vi "GDSIconEditor_GlyphEditorDialog.vi"(8 "error in (no error)":errorcluster, 11 "IconInfo":T3={"HeaderIcon"=[], "RowStart(0)"=0, "ImageRows(32)"=32, "FrameThickness(1)"=1, "FrameColor"=0, "IconTextDataType"={"Text"="", "Allow Only Capital Chars"=FALSE, "Compression"=enum."Auto", "Alignment"=enum."Center"}, "BodyTextColor"=0, "BodyBackgroundColor"=0, "BodyIconHeight"=0, "BodyIconWidth"=0, "HeaderBackgroundColor"=0, "BodyIcon"=[[0, 0, 0, 0, 0, 0, 0, 0, 0, 0, 255, 255, 0, 0, 255, 0, 0, 0, 255, 0, 0, 0, 0, 0, 0, 0, 0, 0, 0, 0], [0, 0, 0, 0, 0, 0, 0, 0, 0, 255, 0, 0, 255, 0, 255, 0, 0, 0, 255, 0, 0, 0, 0, 0, 0, 0, 0, 0, 0, 0], [0, 0, 0, 0, 0, 0, 0, 0, 0, 255, 255, 255, 255, 0, 255, 0, 0, 0, 255, 0, 0, 0, 0, 0, 0, 0, 0, 0, 0, 0], [0, 0, 0, 0, 0, 0, 0, 0, 0, 255, 0, 0, 255, 0, 255, 0, 0, 0, 255, 0, 0, 0, 0, 0, 0, 0, 0, 0, 0, 0], [0, 0, 0, 0, 0, 0, 0, 0, 0, 255, 0, 0, 255, 0, 255, 255, 255, 0, 255, 255, 255, 0, 0, 0, 0, 0, 0, 0, 0, 0], [0, 0, 255, 0, 0, 0, 255, 0, 0, 255, 255, 0, 0, 255, 0, 0, 255, 0, 255, 255, 0, 255, 255, 0, 0, 0, 255, 255, 0, 0], [0, 255, 0, 255, 0, 255, 0, 255, 0, 255, 0, 255, 0, 255, 255, 0, 255, 0, 255, 0, 0, 255, 0, 255, 0, 255, 0, 0, 0, 0], [0, 255, 0, 0, 0, 255, 0, 255, 0, 255, 255, 0, 0, 255, 0, 255, 255, 0, 255, 255, 0, 255, 255, 0, 0, 0, 255, 0, 0, 0], [0, 255, 0, 255, 0, 255, 0, 255, 0, 255, 0, 255, 0, 255, 0, 0, 255, 0, 255, 0, 0, 255, 0, 255, 0, 0, 0, 255, 0, 0], [0, 0, 255, 0, 0, 0, 255, 0, 0, 255, 0, 255, 0, 255, 0, 0, 255, 0, 255, 255, 0, 255, 0, 255, 0, 255, 255, 0, 0, 0], [0, 255, 0, 0, 0, 255, 0, 0, 255, 0, 0, 255, 0, 255, 0, 0, 255, 0, 255, 255, 0, 0, 255, 0, 0, 255, 255, 255, 0, 255], [255, 0, 255, 0, 255, 0, 255, 0, 255, 255, 0, 255, 0, 255, 255, 0, 255, 0, 255, 0, 0, 255, 0, 255, 0, 0, 255, 0, 0, 255], [255, 0, 0, 0, 255, 0, 255, 0, 255, 0, 255, 255, 0, 255, 0, 255, 255, 0, 255, 255, 0, 255, 0, 0, 0, 0, 255, 0, 0, 255], [255, 0, 255, 0, 255, 0, 255, 0, 255, 0, 0, 255, 0, 255, 0, 0, 255, 0, 255, 0, 0, 255, 0, 255, 0, 0, 255, 0, 0, 255], [0, 255, 0, 0, 0, 255, 0, 0, 255, 0, 0, 255, 0, 255, 0, 0, 255, 0, 255, 255, 0, 0, 255, 0, 0, 0, 255, 0, 0, 255], [0, 0, 0, 0, 0, 0, 0, 0, 0, 0, 0, 0, 0, 0, 255, 0, 0, 0, 0, 0, 0, 0, 0, 0, 0, 0, 0, 0, 0, 0], [0, 0, 0, 0, 0, 0, 0, 0, 0, 0, 0, 0, 0, 255, 0, 0, 0, 0, 0, 0, 0, 0, 0, 0, 0, 0, 0, 0, 0, 0], [0, 0, 0, 0, 0, 0, 0, 0, 0, 0, 0, 0, 0, 255, 255, 0, 0, 0, 0, 0, 0, 0, 0, 0, 0, 0, 0, 0, 0, 0], [0, 0, 0, 0, 0, 0, 0, 0, 0, 0, 0, 0, 0, 255, 0, 255, 0, 0, 0, 0, 0, 0, 0, 0, 0, 0, 0, 0, 0, 0], [0, 0, 0, 0, 0, 0, 0, 0, 0, 0, 0, 0, 0, 0, 255, 0, 0, 0, 0, 0, 0, 0, 0, 0, 0, 0, 0, 0, 0, 0], [0, 0, 0, 0, 0, 0, 0, 0, 0, 0, 0, 0, 0, 0, 0, 0, 0, 0, 0, 0, 0, 0, 0, 0, 0, 0, 0, 0, 0, 0], [0, 0, 0, 0, 0, 0, 0, 0, 0, 0, 0, 0, 0, 0, 0, 0, 0, 0, 0, 0, 0, 0, 0, 0, 0, 0, 0, 0, 0, 0]], "Offset"={"X"=0, "Y"=0}, "CurrentIcon"={"BgIcon"=[], "BgIconOffset"={"X"=0, "Y"=0}, "BgIconMask"=[], "ColorsOkayforiconToBeOnTopOf"=[]}} {"HeaderIcon" format="%x"}) -> (0 "error out":errorcluster, 1 "Icon exist":bool, 2 "CurrentIcon":T2, 3 "Cancelled":bool, 5 "Offset":cluster{"X":i32, "Y":i32}, 7 "BodyIcon":u8[][](array[numeric]))   [LabVIEW 2020]
uses:
  <resource>/Framework/Providers/Open_GDS/ClassProviders/Common/IconEditor/private/GDSIconEditor_IconDialog_Input.vi
  <resource>/Framework/Providers/Open_GDS/ClassProviders/Common/LvIcon_class/subvis/GDSLvIcon_TextDataType.ctl
  <resource>/Framework/Providers/Open_GDS/ClassProviders/Common/LvIcon_class/GDSLvIcon_WordCompressionType.ctl
  <resource>/Framework/Providers/Open_GDS/ClassProviders/Common/LvIcon_class/GDSLvIcon_TextAlignment.ctl
  <vilib>/picture/picture.llb/imagedata.ctl
  <vilib>/Utility/miscctls.llb/LVPoint32TypeDef.ctl
  <vilib>/Utility/miscctls.llb/LVPointTypeDef.ctl
  <vilib>/Utility/miscctls.llb/LVPositionTypeDef.ctl
panel:
  in  "Positon":T1(ring)
  in  "Relative to Error terminals":bool
  out "_IconPreview 2":picture caption="Icon Preview"
  out "_After 2":picture caption="New"
  in  "Remove Configuration":bool
  in  "Add Configuration":bool
  in  "Quick selection icons":i32(listbox)
  out "_IconPreview":picture caption="Icon Preview"
  in  "FloodFillMask":bool
  out "_After":picture caption="New"
  out "_IconName":string
  out "DragIcon":picture
  out "ProductPicture":picture
  in  "_IconSearchText":string caption="Icon search text"
  in  "_Manage":bool
  in  "_Folders":u16(ring) caption="Folders" items=["<All icons>", "C:\\Program Files (x86)\\National Instruments\\LabVIEW 2020\\resource\\Framework\\Providers\\Icons", "C:\\Program Files (x86)\\National Instruments\\LabVIEW 2020\\resource\\Framework\\Providers\\Open_GDS\\Glyphs", "C:\\Program Files (x86)\\National Instruments\\LabVIEW 2020\\resource\\Framework\\Providers\\Open_GDS\\Icons", "C:\\Users\\mikael.holmstrom\\Documents\\LabVIEW Data\\Glyphs"]
  out "Icons":picture
  in  "_HelpCreateClass":bool
  in  "_Cancel":bool
  in  "Accept":bool
  # "Drag icon into preview wndow"
  # "User arrow keys to move text,\nor drar the text to move it."
  # "User arrow keys to move text,\nor drar the text to move it."
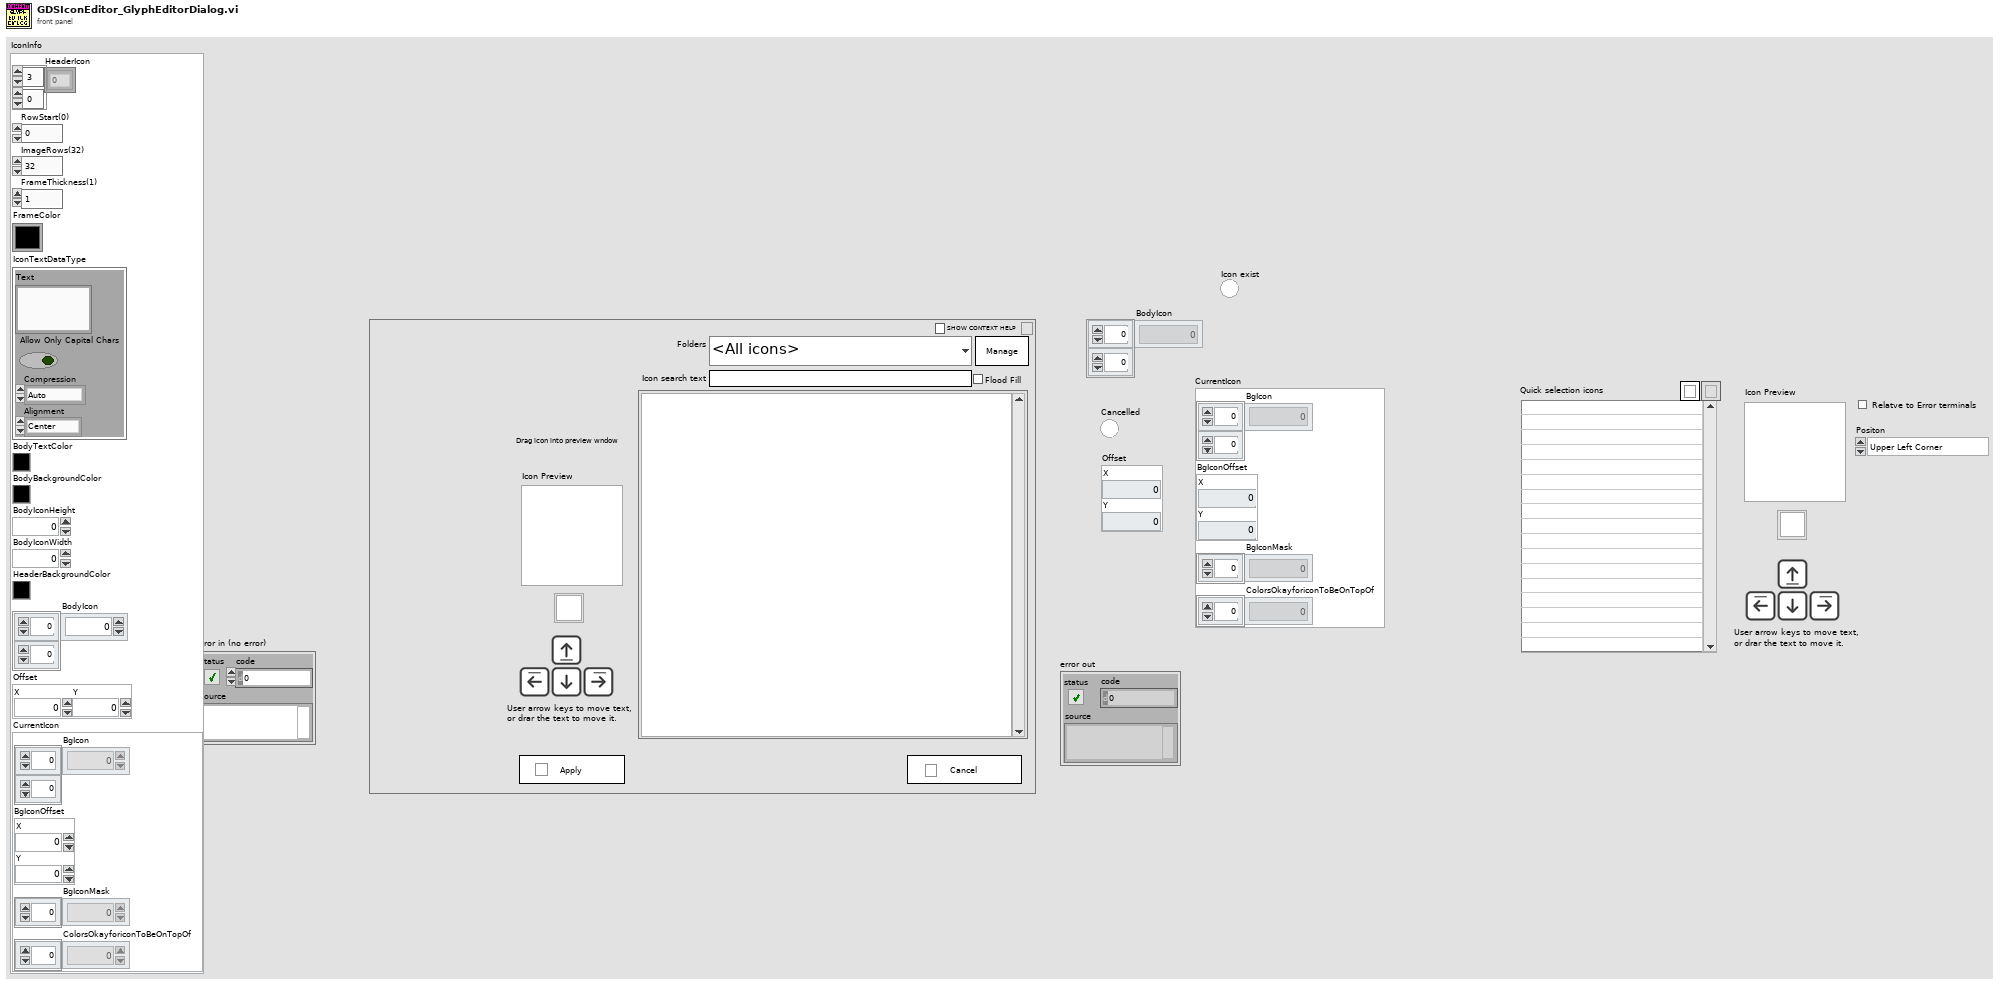
[diagram p1: front panel]
types:
  T1 = enum16{"Upper Left Corner", "Error In Terminal (Center)"}
  T2 = cluster{"BgIcon":u8[][], "BgIconOffset":cluster{"X":i32, "Y":i32}, "BgIconMask":u8[], "ColorsOkayforiconToBeOnTopOf":u8[]}
  T3 = typedef "GDSIconEditor_IconDialog_Input.vi" = cluster{"HeaderIcon":u8[][], "RowStart(0)":i32, "ImageRows(32)":i32, "FrameThickness(1)":u32, "FrameColor":u32, "IconTextDataType":T4, "BodyTextColor":u32, "BodyBackgroundColor":u32, "BodyIconHeight":i32, "BodyIconWidth":i32, "HeaderBackgroundColor":u32, "BodyIcon":u8[][], "Offset":cluster{"X":i32, "Y":i32}, "CurrentIcon":cluster{"BgIcon":u8[][], "BgIconOffset":cluster{"X":i32, "Y":i32}, "BgIconMask":u8[], "ColorsOkayforiconToBeOnTopOf":u8[]}}
  T4 = typedef "GDSLvIcon_TextDataType.ctl" = cluster{"Text":string, "Allow Only Capital Chars":bool, "Compression":T5, "Alignment":T6}
  T5 = typedef "GDSLvIcon_WordCompressionType.ctl" = enum16{"Auto", "On", "Off"}
  T6 = typedef "GDSLvIcon_TextAlignment.ctl" = enum16{"Center", "Left", "Right"}
  T7 = typedef "imagedata.ctl" = cluster{"image type":i32, "image depth":i32, "image":u8[], "mask":u8[], "colors":u32[], "Rectangle":cluster{"left":i16, "top":i16, "right":i16, "bottom":i16}}
  T8 = typedef "LVPoint32TypeDef.ctl" = cluster{"Horizontal":i32, "Vertical":i32}
  T9 = cluster{"Icons":T7[], "Folders":path[], "IconPaths":cluster{i32, "path out":path}[], "IconPos":cluster{"left":i16, "top":i16, "right":i16, "bottom":i16}[], "IconNames":string[], "DraggingIcon":bool, "DraggingText":bool, "IconSelected":i32, "IconDropped":i32, "BgIcon":u8[][], "BgIconOffset":cluster{"X":i32, "Y":i32}, "BgIconMask":u8[], "IconOut":u8[][], "ConnectorPaneHeight":i32[], "BodyIcon":u8[][], "Cancelled":bool, "StartTextDraggingPos":T8, "OldOffset":cluster{"X":i32, "Y":i32}, "TextBounds":cluster{"FirstRow":i32, "FirstColumn":i32, "LastRow":i32, "LastColumn":i32}, "Moving":bool, "Icon exist":bool, "IconInfo":T3}
  T10 = typedef "LVPointTypeDef.ctl" = cluster{"Horizontal":i16, "Vertical":i16}
  T11 = typedef "LVPositionTypeDef.ctl" = cluster{"Left":i32, "Top":i32}
  T12 = typedef "LVBoundsTypeDef.ctl" = cluster{"Width":u32, "Height":u32}
  T13 = cluster{"left":i16, "top":i16, "right":i16, "bottom":i16}
  T14 = cluster{"left":i16, "top":i16, "right":i16, "bottom":i16}[]
  T15 = typedef "LVMouseTypeDef.ctl" = cluster{"Mouse Position":cluster{"X":i32, "Y":i32}, "Mouse Modifiers":cluster{"Button Down":bool, "Shift Mod":bool, "Menu Mod":bool, "Option Mod":bool}}
  T16 = cluster{"FirstRow":i32, "FirstColumn":i32, "LastRow":i32, "LastColumn":i32}
  T17 = typedef "eventvkey.ctl" = enum16{"ASCII", "Enter", "Return", "Shift", "Ctrl", "Alt", "Cmd", "Opt", "Caps", "NumLock", "Clear", "Break", "Up", "Down", "Left", "Right", "Insert", "Delete", "Home", "End", "PageUp", "PageDown", "Escape", "Help", "Pause", "ScrollLock", "F1", "F2", "F3", "F4", "F5", "F6", "F7", "F8", "F9", "F10", "F11", "F12", "F13", "F14", "F15", "F16", "F17", "F18", "F19", "F20", "F21", "F22", "F23", "F24", "Play", "VolumeUp", "VolumeDown", "Mute", "Two Byte Char"}
  T18 = cluster{"Shift":bool, "Ctrl":bool, "Alt":bool, "Cmd":bool, "Opt":bool}
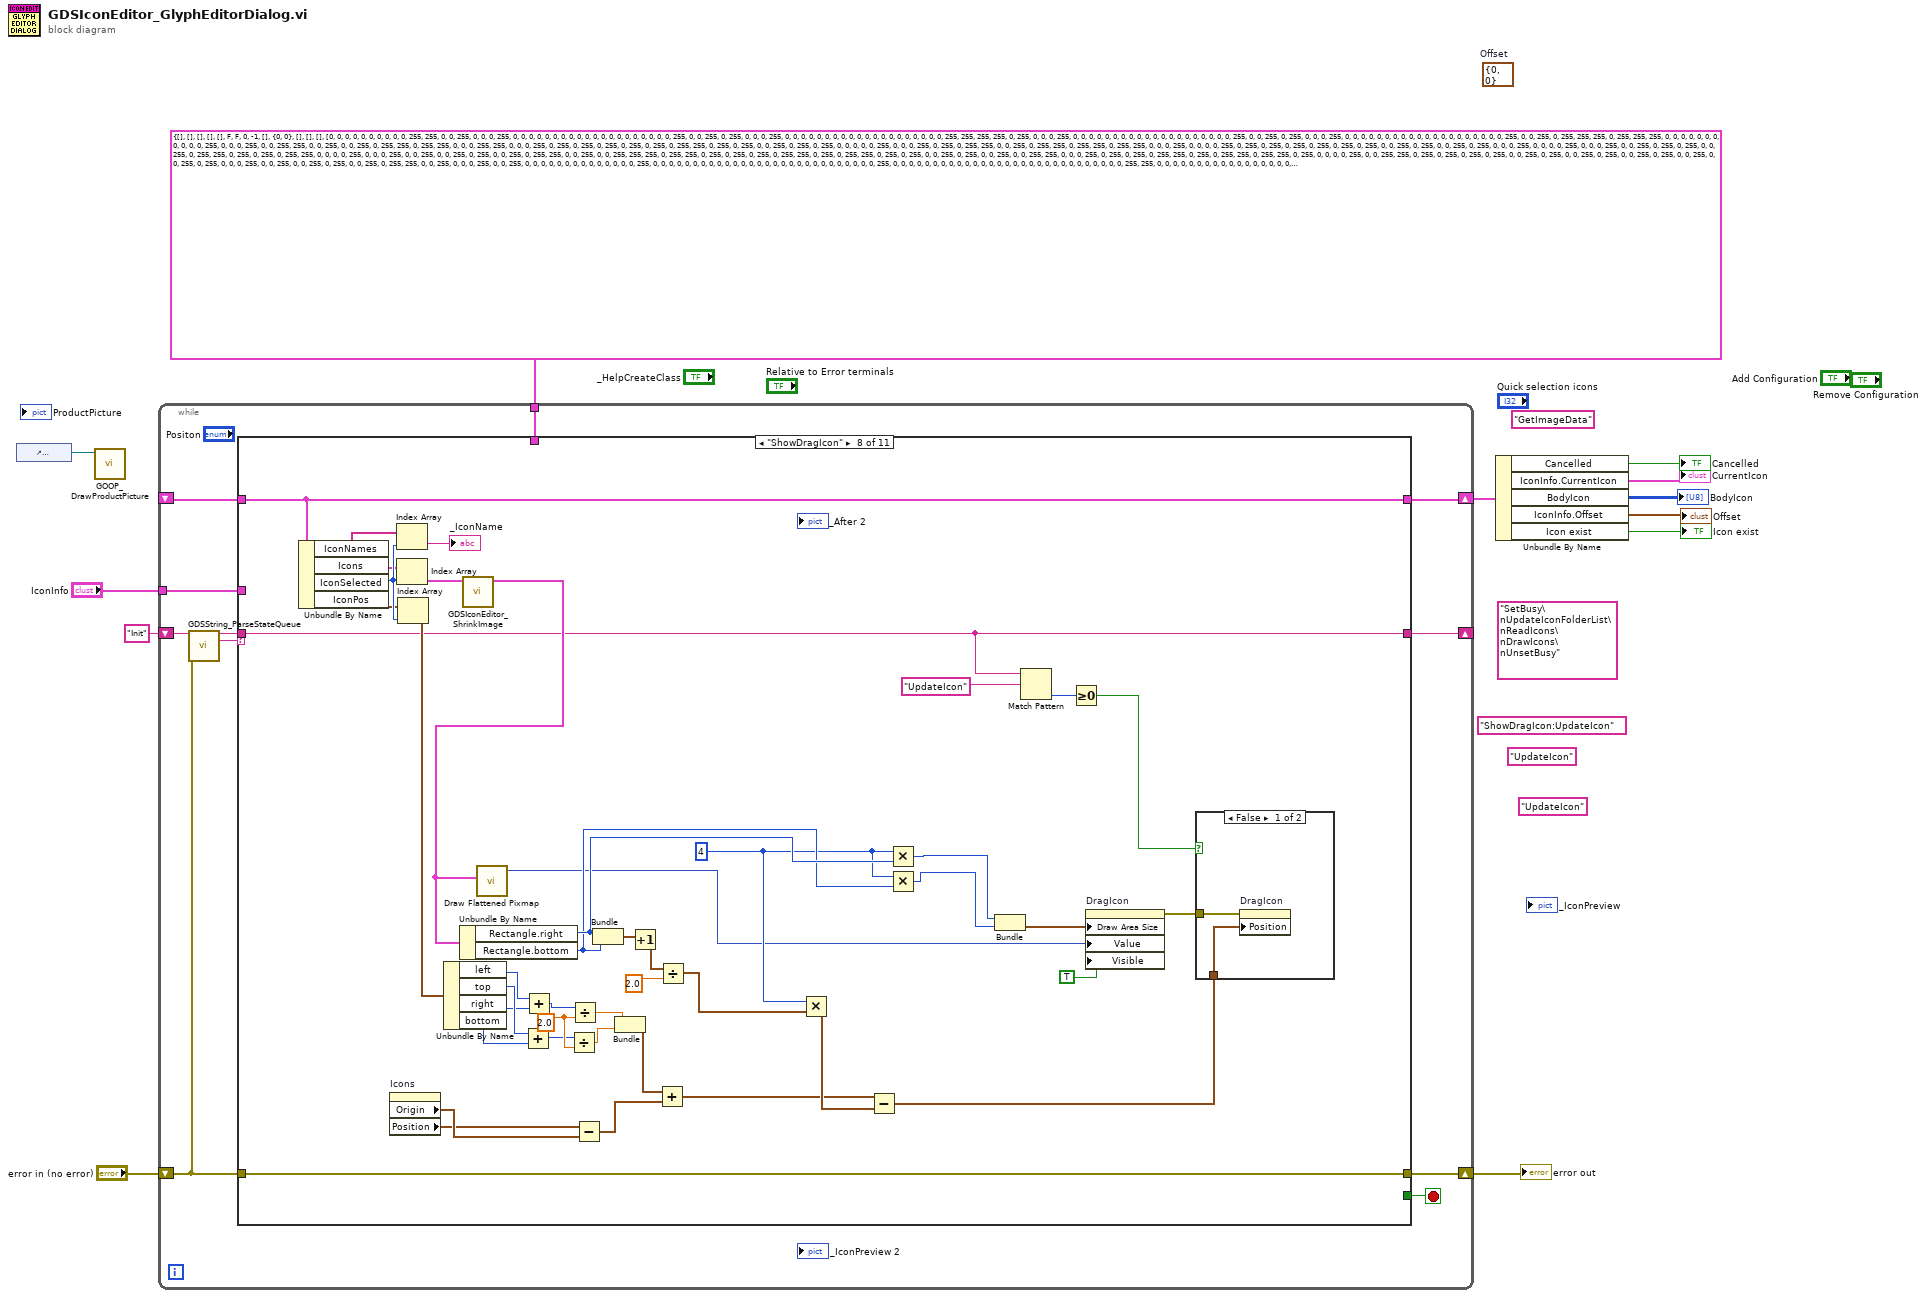
[diagram p0: block diagram]
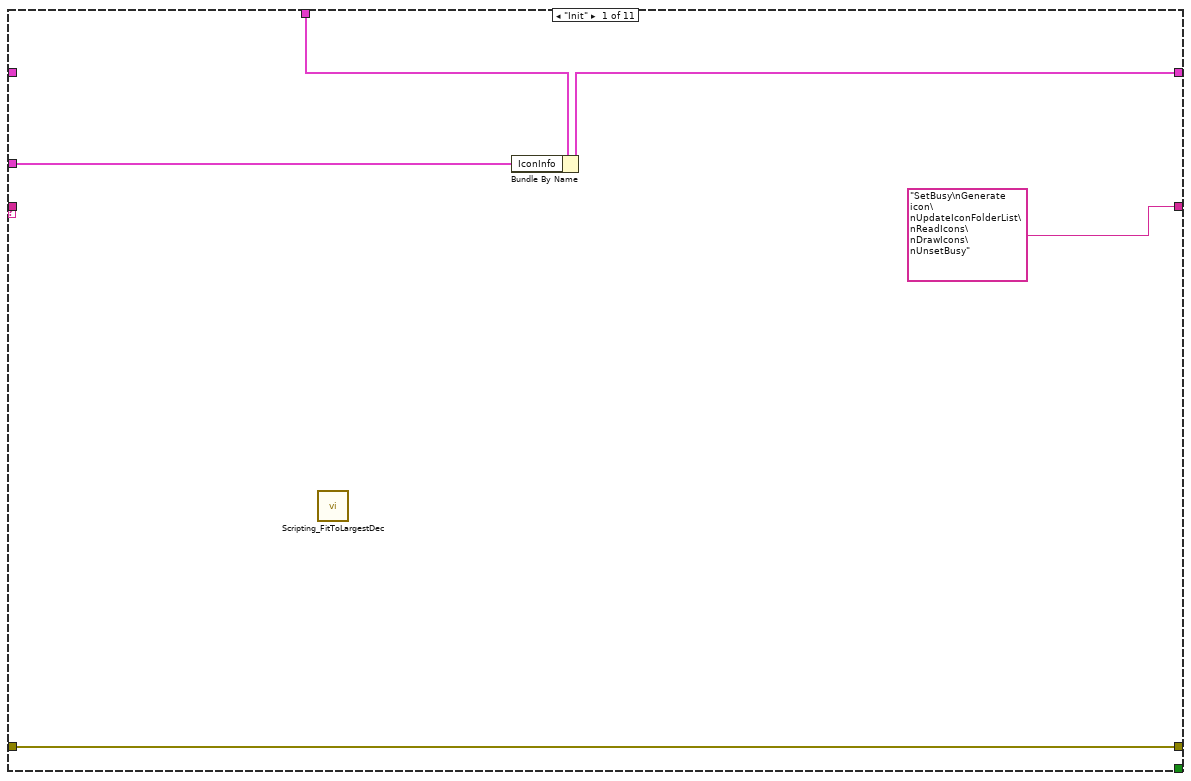
[diagram p2: hidden frame]
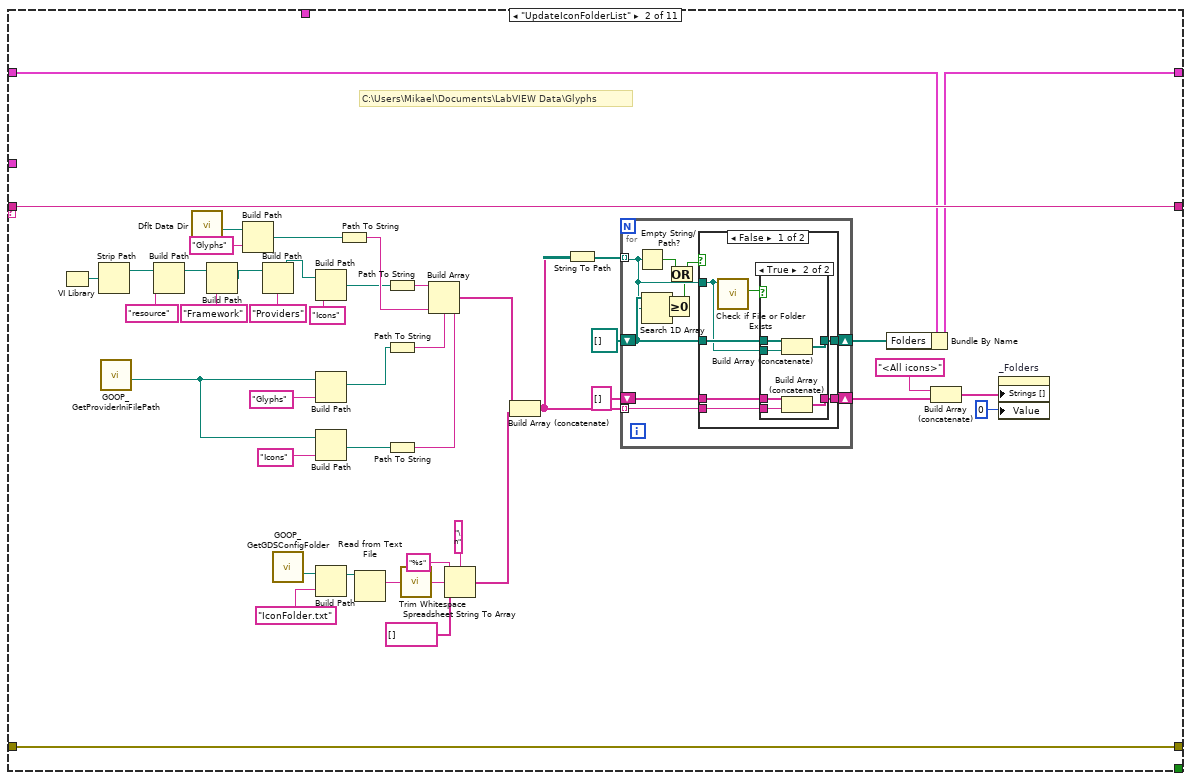
[diagram p3: hidden frame]
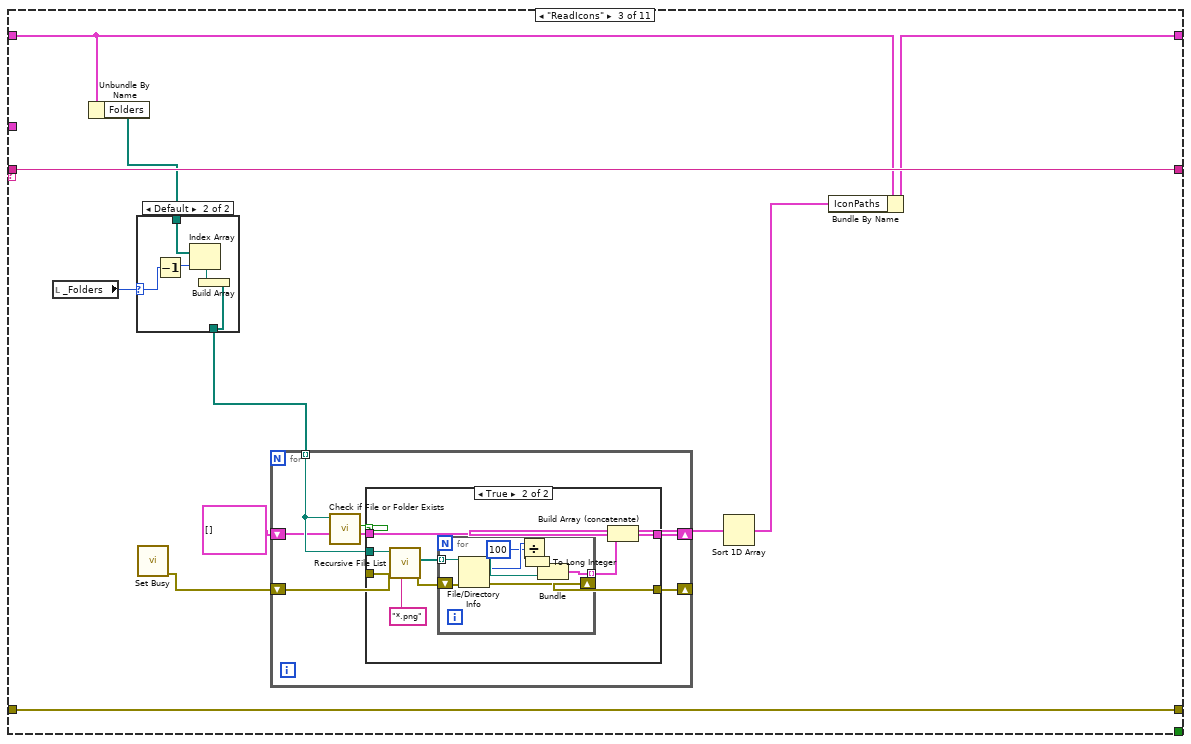
[diagram p6: hidden frame]
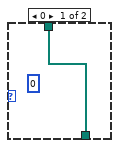
[diagram p7: hidden frame]
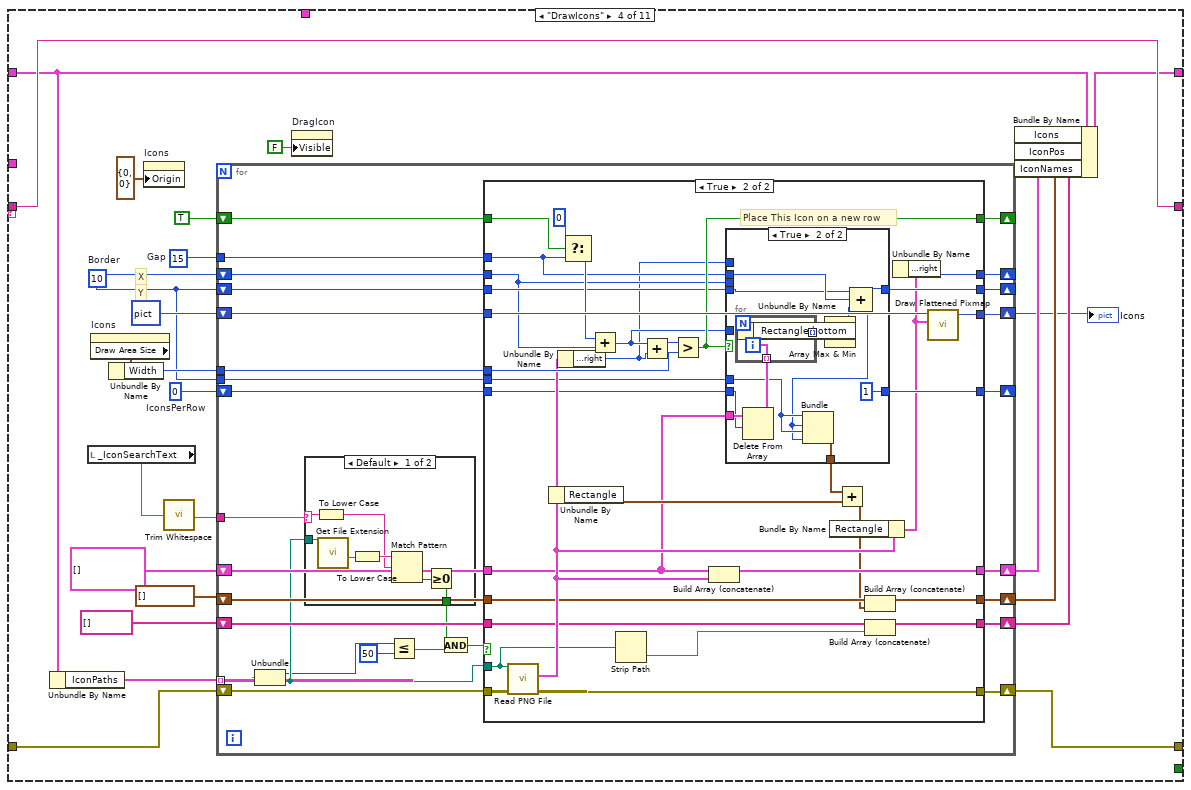
[diagram p9: hidden frame]
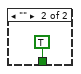
[diagram p10: hidden frame]
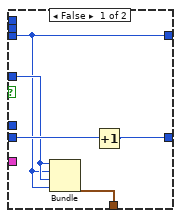
[diagram p12: hidden frame]
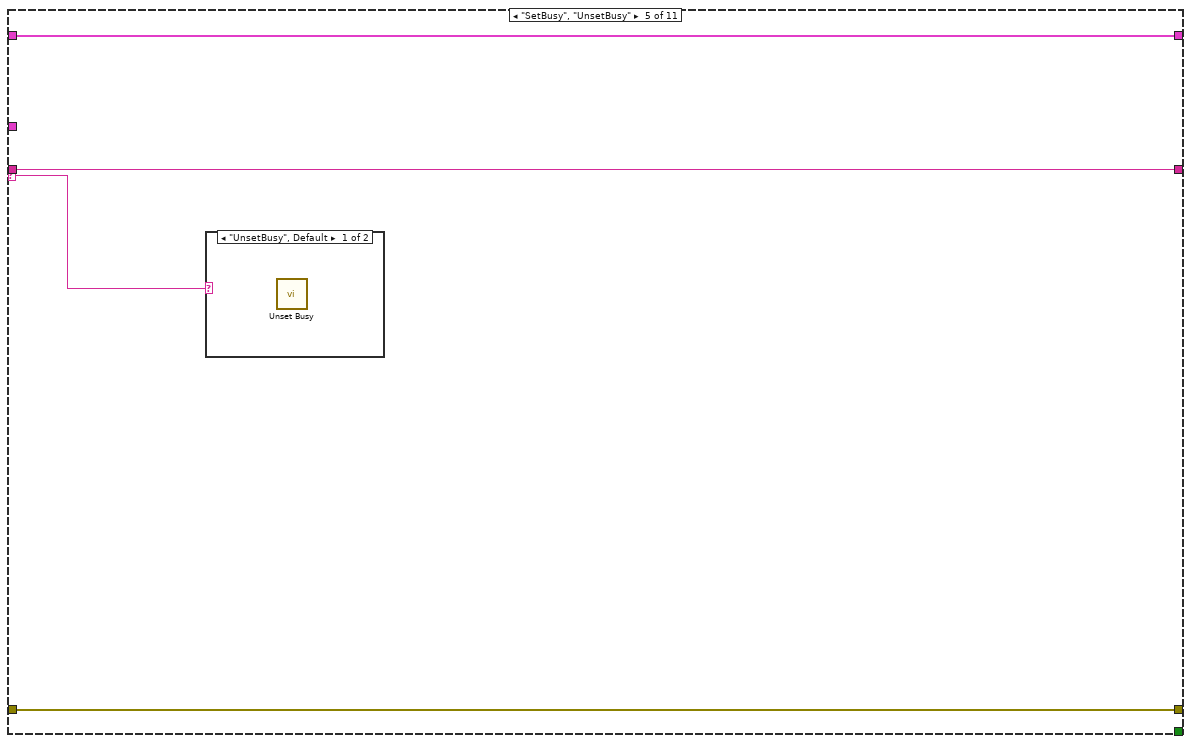
[diagram p13: hidden frame]
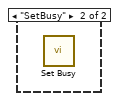
[diagram p14: hidden frame]
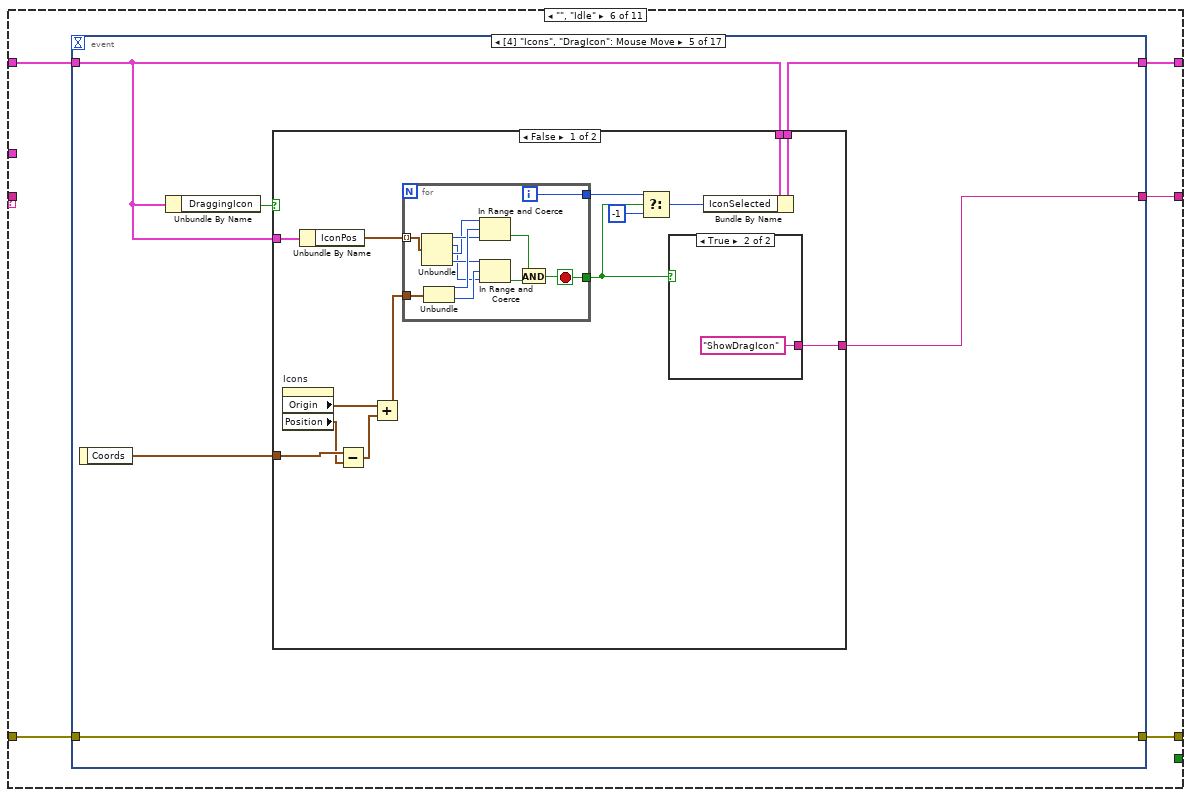
[diagram p15: hidden frame]
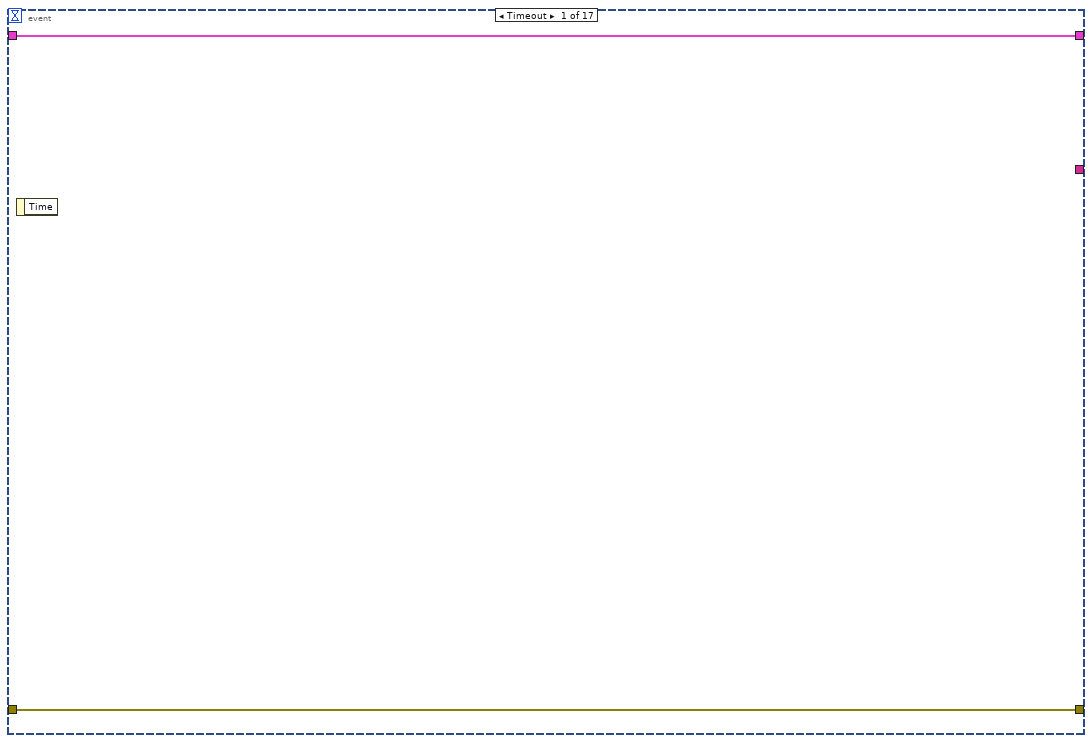
[diagram p16: hidden frame]
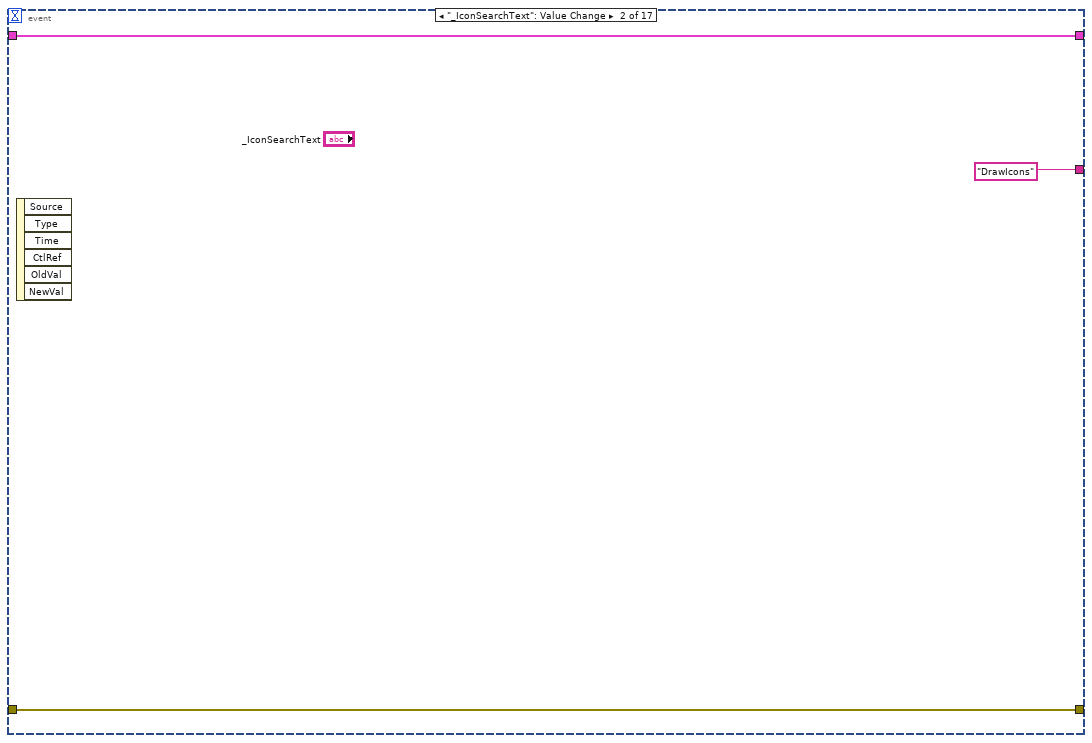
[diagram p17: hidden frame]
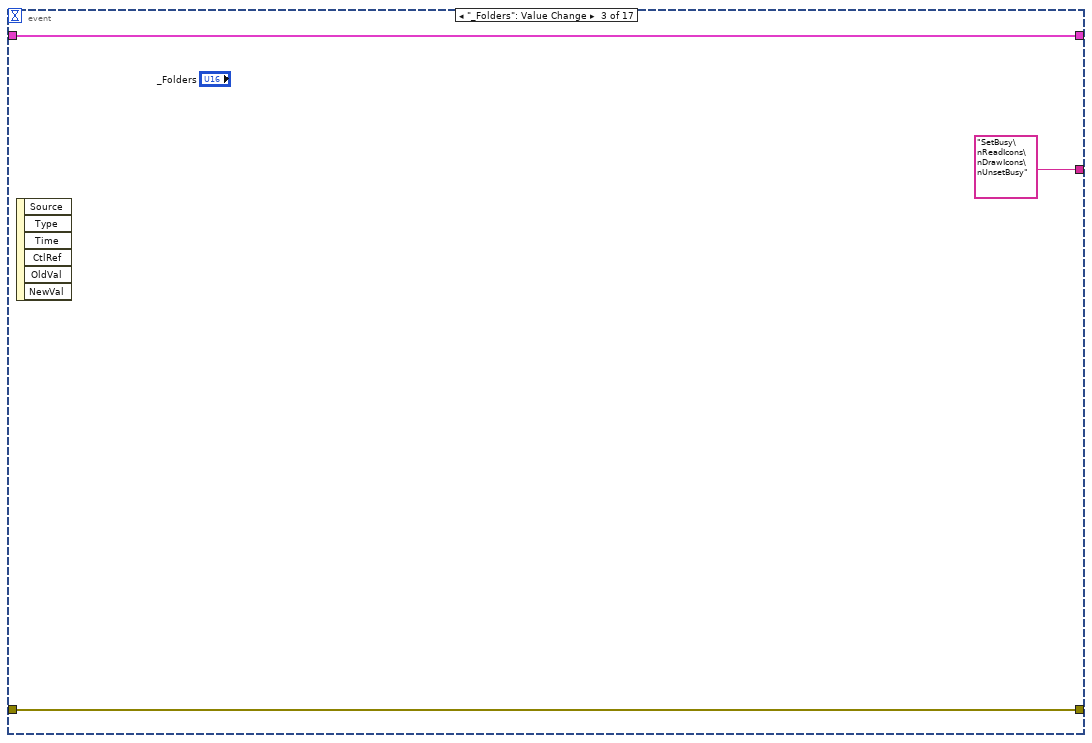
[diagram p18: hidden frame]
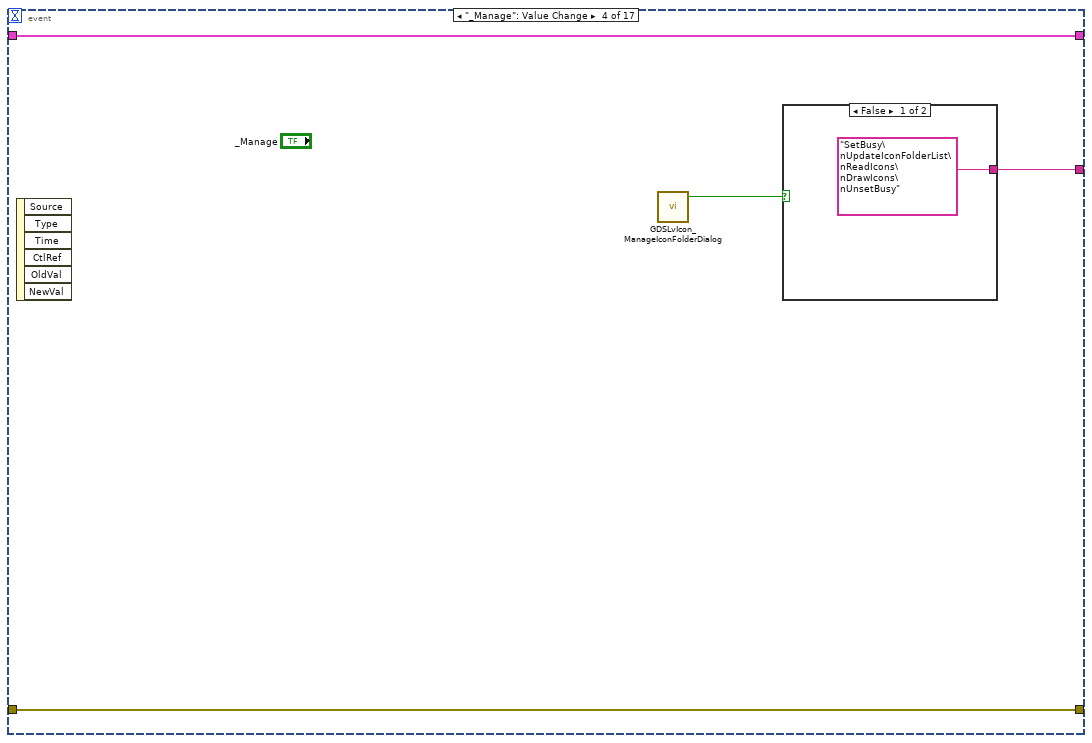
[diagram p19: hidden frame]
diagram:
  (unwired) cluster{"X":i32, "Y":i32} {"X"=0, "Y"=0}  # Offset
  (unwired) "UpdateIcon" ("y")
  (unwired) "GetImageData" ("y")
  (unwired) "ShowDragIcon:UpdateIcon" ("y")
  (unwired) "UpdateIcon" ("t")
  (unwired) "SetBusy\nUpdateIconFolderList\nReadIcons\nDrawIcons\nUnsetBusy"
  n1 = control-ref of="ProductPicture"() -> (w1:refnum<vi>)
  n2 = call <resource>:"GOOP_DrawProductPicture.vi"("ProductPictureControl"=w1) -> ()  [unwired: 10 in, 1 out]
  n3 = while {
    shift-right: [w22] -> w8
    shift-left: _ -> [w17]
    tunnel: T9 {"Icons"=[], "Folders"=[], "IconPaths"=[], "IconPos"=[], "IconNames"=[], "DraggingIcon"=FALSE, "DraggingText"=FALSE, "IconSelected"=0, "IconDropped"=-1, "BgIcon"=[], "BgIconOffset"={"X"=0, "Y"=0}, "BgIconMask"=[], "IconOut"=[], "ConnectorPaneHeight"=[], "BodyIcon"=[[0, 0, 0, 0, 0, 0, 0, 0, 0, 0, 255, 255, 0, 0, 255, 0, 0, 0, 255, 0, 0, 0, 0, 0, 0, 0, 0, 0, 0, 0], [0, 0, 0, 0, 0, 0, 0, 0, 0, 255, 0, 0, 255, 0, 255, 0, 0, 0, 255, 0, 0, 0, 0, 0, 0, 0, 0, 0, 0, 0], [0, 0, 0, 0, 0, 0, 0, 0, 0, 255, 255, 255, 255, 0, 255, 0, 0, 0, 255, 0, 0, 0, 0, 0, 0, 0, 0, 0, 0, 0], [0, 0, 0, 0, 0, 0, 0, 0, 0, 255, 0, 0, 255, 0, 255, 0, 0, 0, 255, 0, 0, 0, 0, 0, 0, 0, 0, 0, 0, 0], [0, 0, 0, 0, 0, 0, 0, 0, 0, 255, 0, 0, 255, 0, 255, 255, 255, 0, 255, 255, 255, 0, 0, 0, 0, 0, 0, 0, 0, 0], [0, 0, 255, 0, 0, 0, 255, 0, 0, 255, 255, 0, 0, 255, 0, 0, 255, 0, 255, 255, 0, 255, 255, 0, 0, 0, 255, 255, 0, 0], [0, 255, 0, 255, 0, 255, 0, 255, 0, 255, 0, 255, 0, 255, 255, 0, 255, 0, 255, 0, 0, 255, 0, 255, 0, 255, 0, 0, 0, 0], [0, 255, 0, 0, 0, 255, 0, 255, 0, 255, 255, 0, 0, 255, 0, 255, 255, 0, 255, 255, 0, 255, 255, 0, 0, 0, 255, 0, 0, 0], [0, 255, 0, 255, 0, 255, 0, 255, 0, 255, 0, 255, 0, 255, 0, 0, 255, 0, 255, 0, 0, 255, 0, 255, 0, 0, 0, 255, 0, 0], [0, 0, 255, 0, 0, 0, 255, 0, 0, 255, 0, 255, 0, 255, 0, 0, 255, 0, 255, 255, 0, 255, 0, 255, 0, 255, 255, 0, 0, 0], [0, 255, 0, 0, 0, 255, 0, 0, 255, 0, 0, 255, 0, 255, 0, 0, 255, 0, 255, 255, 0, 0, 255, 0, 0, 255, 255, 255, 0, 255], [255, 0, 255, 0, 255, 0, 255, 0, 255, 255, 0, 255, 0, 255, 255, 0, 255, 0, 255, 0, 0, 255, 0, 255, 0, 0, 255, 0, 0, 255], [255, 0, 0, 0, 255, 0, 255, 0, 255, 0, 255, 255, 0, 255, 0, 255, 255, 0, 255, 255, 0, 255, 0, 0, 0, 0, 255, 0, 0, 255], [255, 0, 255, 0, 255, 0, 255, 0, 255, 0, 0, 255, 0, 255, 0, 0, 255, 0, 255, 0, 0, 255, 0, 255, 0, 0, 255, 0, 0, 255], [0, 255, 0, 0, 0, 255, 0, 0, 255, 0, 0, 255, 0, 255, 0, 0, 255, 0, 255, 255, 0, 0, 255, 0, 0, 0, 255, 0, 0, 255], [0, 0, 0, 0, 0, 0, 0, 0, 0, 0, 0, 0, 0, 0, 255, 0, 0, 0, 0, 0, 0, 0, 0, 0, 0, 0, 0, 0, 0, 0], [0, 0, 0, 0, 0, 0, 0, 0, 0, 0, 0, 0, 0, 255, 0, 0, 0, 0, 0, 0, 0, 0, 0, 0, 0, 0, 0, 0, 0, 0], [0, 0, 0, 0, 0, 0, 0, 0, 0, 0, 0, 0, 0, 255, 255, 0, 0, 0, 0, 0, 0, 0, 0, 0, 0, 0, 0, 0, 0, 0], [0, 0, 0, 0, 0, 0, 0, 0, 0, 0, 0, 0, 0, 255, 0, 255, 0, 0, 0, 0, 0, 0, 0, 0, 0, 0, 0, 0, 0, 0], [0, 0, 0, 0, 0, 0, 0, 0, 0, 0, 0, 0, 0, 0, 255, 0, 0, 0, 0, 0, 0, 0, 0, 0, 0, 0, 0, 0, 0, 0], [0, 0, 0, 0, 0, 0, 0, 0, 0, 0, 0, 0, 0, 0, 0, 0, 0, 0, 0, 0, 0, 0, 0, 0, 0, 0, 0, 0, 0, 0], [0, 0, 0, 0, 0, 0, 0, 0, 0, 0, 0, 0, 0, 0, 0, 0, 0, 0, 0, 0, 0, 0, 0, 0, 0, 0, 0, 0, 0, 0]], "Cancelled"=FALSE, "StartTextDraggingPos"={"Horizontal"=0, "Vertical"=0}, "OldOffset"={"X"=0, "Y"=0}, "TextBounds"={"FirstRow"=2, "FirstColumn"=1, "LastRow"=6, "LastColumn"=27}, "Moving"=FALSE, "Icon exist"=FALSE, "IconInfo"={"HeaderIcon"=[], "RowStart(0)"=0, "ImageRows(32)"=32, "FrameThickness(1)"=1, "FrameColor"=0, "IconTextDataType"={"Text"="", "Allow Only Capital Chars"=FALSE, "Compression"=enum."Auto", "Alignment"=enum."Center"}, "BodyTextColor"=0, "BodyBackgroundColor"=0, "BodyIconHeight"=0, "BodyIconWidth"=0, "HeaderBackgroundColor"=0, "BodyIcon"=[[0, 0, 0, 0, 0, 0, 0, 0, 0, 0, 255, 255, 0, 0, 255, 0, 0, 0, 255, 0, 0, 0, 0, 0, 0, 0, 0, 0, 0, 0], [0, 0, 0, 0, 0, 0, 0, 0, 0, 255, 0, 0, 255, 0, 255, 0, 0, 0, 255, 0, 0, 0, 0, 0, 0, 0, 0, 0, 0, 0], [0, 0, 0, 0, 0, 0, 0, 0, 0, 255, 255, 255, 255, 0, 255, 0, 0, 0, 255, 0, 0, 0, 0, 0, 0, 0, 0, 0, 0, 0], [0, 0, 0, 0, 0, 0, 0, 0, 0, 255, 0, 0, 255, 0, 255, 0, 0, 0, 255, 0, 0, 0, 0, 0, 0, 0, 0, 0, 0, 0], [0, 0, 0, 0, 0, 0, 0, 0, 0, 255, 0, 0, 255, 0, 255, 255, 255, 0, 255, 255, 255, 0, 0, 0, 0, 0, 0, 0, 0, 0], [0, 0, 255, 0, 0, 0, 255, 0, 0, 255, 255, 0, 0, 255, 0, 0, 255, 0, 255, 255, 0, 255, 255, 0, 0, 0, 255, 255, 0, 0], [0, 255, 0, 255, 0, 255, 0, 255, 0, 255, 0, 255, 0, 255, 255, 0, 255, 0, 255, 0, 0, 255, 0, 255, 0, 255, 0, 0, 0, 0], [0, 255, 0, 0, 0, 255, 0, 255, 0, 255, 255, 0, 0, 255, 0, 255, 255, 0, 255, 255, 0, 255, 255, 0, 0, 0, 255, 0, 0, 0], [0, 255, 0, 255, 0, 255, 0, 255, 0, 255, 0, 255, 0, 255, 0, 0, 255, 0, 255, 0, 0, 255, 0, 255, 0, 0, 0, 255, 0, 0], [0, 0, 255, 0, 0, 0, 255, 0, 0, 255, 0, 255, 0, 255, 0, 0, 255, 0, 255, 255, 0, 255, 0, 255, 0, 255, 255, 0, 0, 0], [0, 255, 0, 0, 0, 255, 0, 0, 255, 0, 0, 255, 0, 255, 0, 0, 255, 0, 255, 255, 0, 0, 255, 0, 0, 255, 255, 255, 0, 255], [255, 0, 255, 0, 255, 0, 255, 0, 255, 255, 0, 255, 0, 255, 255, 0, 255, 0, 255, 0, 0, 255, 0, 255, 0, 0, 255, 0, 0, 255], [255, 0, 0, 0, 255, 0, 255, 0, 255, 0, 255, 255, 0, 255, 0, 255, 255, 0, 255, 255, 0, 255, 0, 0, 0, 0, 255, 0, 0, 255], [255, 0, 255, 0, 255, 0, 255, 0, 255, 0, 0, 255, 0, 255, 0, 0, 255, 0, 255, 0, 0, 255, 0, 255, 0, 0, 255, 0, 0, 255], [0, 255, 0, 0, 0, 255, 0, 0, 255, 0, 0, 255, 0, 255, 0, 0, 255, 0, 255, 255, 0, 0, 255, 0, 0, 0, 255, 0, 0, 255], [0, 0, 0, 0, 0, 0, 0, 0, 0, 0, 0, 0, 0, 0, 255, 0, 0, 0, 0, 0, 0, 0, 0, 0, 0, 0, 0, 0, 0, 0], [0, 0, 0, 0, 0, 0, 0, 0, 0, 0, 0, 0, 0, 255, 0, 0, 0, 0, 0, 0, 0, 0, 0, 0, 0, 0, 0, 0, 0, 0], [0, 0, 0, 0, 0, 0, 0, 0, 0, 0, 0, 0, 0, 255, 255, 0, 0, 0, 0, 0, 0, 0, 0, 0, 0, 0, 0, 0, 0, 0], [0, 0, 0, 0, 0, 0, 0, 0, 0, 0, 0, 0, 0, 255, 0, 255, 0, 0, 0, 0, 0, 0, 0, 0, 0, 0, 0, 0, 0, 0], [0, 0, 0, 0, 0, 0, 0, 0, 0, 0, 0, 0, 0, 0, 255, 0, 0, 0, 0, 0, 0, 0, 0, 0, 0, 0, 0, 0, 0, 0], [0, 0, 0, 0, 0, 0, 0, 0, 0, 0, 0, 0, 0, 0, 0, 0, 0, 0, 0, 0, 0, 0, 0, 0, 0, 0, 0, 0, 0, 0], [0, 0, 0, 0, 0, 0, 0, 0, 0, 0, 0, 0, 0, 0, 0, 0, 0, 0, 0, 0, 0, 0, 0, 0, 0, 0, 0, 0, 0, 0]], "Offset"={"X"=0, "Y"=0}, "CurrentIcon"={"BgIcon"=[], "BgIconOffset"={"X"=0, "Y"=0}, "BgIconMask"=[], "ColorsOkayforiconToBeOnTopOf"=[]}}} -> [w21]
    shift-right: [w18] -> _
    shift-left: "Init" ("Remaining States") -> [w20]
    shift-right: [w16] -> w10
    shift-left: "error in (no error)" -> [w15]
    tunnel: "IconInfo" -> [w13]
    stop <- w14 stop-if-true
    n4 = call <resource>:"GDSString_ParseStateQueue.vi"("State Queue"=w20, "Error In (no error)"=w15) -> ("Remaining States"=w19:string, "Current State"=w23:string)  [unwired: 9 in, 3 out]
    n5 = case shown="\"ShowDragIcon\"" w23 {
      selector: w23 -> [_ _ _ _ w265 _ _ _ _ _ _]
      tunnel: [w25 w33 w103 w148 w268 w272 w539 w560 w600 w642 w664] -> w22
      tunnel: w21 -> [w28 _ _ _ _ _ _ _ _ _ _]
      tunnel: w19 -> [_ w34 w111 w149 w267 _ w549 w557 w623 w624 w665]
      tunnel: ["SetBusy\nGenerate icon\nUpdateIconFolderList\nReadIcons\nDrawIcons\nUnsetBusy" w34 w111 w149 w267 w269 w549 w557 w623 w624 w665] -> w18
      tunnel: w17 -> [_ w32 w102 w147 w268 w273 w538 w560 w599 w635 w664]
      tunnel: w15 -> [w27 w73 w110 w144 w266 w271 w548 w596 w605 w636 w663]
      tunnel: [w27 w73 w110 w145 w266 w270 w548 w596 w606 w637 w663] -> w16
      tunnel: [_ _ _ _ _ _ _ _ _ _ TRUE] -> w14
      tunnel: w13 -> [w24 _ _ _ _ _ _ _ _ _ _]
      frame "Init" {
        n6 = call <resource>:"Scripting_FitToLargestDec.vi"() -> ()  [unwired: 6 in, 2 out]
        n7 = Bundle By Name(cluster=w28, "IconInfo"=w24) -> (w25:T9)
      }
      frame "UpdateIconFolderList" {
        # "C:\\Users\\Mikael\\Documents\\LabVIEW Data\\Glyphs"
        n8 = VI Library() -> (path=w62:path)
        n9 = Strip Path(path=w62) -> (stripped path=w50:path)  [unwired: 1 out]
        n10 = call <resource>:"GOOP_GetProviderIniFilePath.vi"() -> ("ProviderMainFolder"=w69:path)  [unwired: 10 in, 1 out]
        n11 = Build Path(base path=w50, name or relative path="resource") -> (appended path=w61:path)
        n12 = call <vilib>:"Dflt Data Dir.vi"() -> ("App:Default Data Directory"=w54:path)
        n13 = Build Path(base path=w61, name or relative path="Framework") -> (appended path=w60:path)
        n14 = Build Path(base path=w54, name or relative path="Glyphs") -> (appended path=w53:path)
        n15 = Build Path(base path=w60, name or relative path="Providers") -> (appended path=w51:path)
        n16 = call <resource>:"GOOP_GetGDSConfigFolder.vi"() -> ("GDSFolderPath"=w35:path)
        n17 = Build Path(base path=w51, name or relative path="Icons") -> (appended path=w65:path)
        n18 = Build Path(base path=w69, name or relative path="Glyphs") -> (appended path=w67:path)
        n19 = Build Path(base path=w69, name or relative path="Icons") -> (appended path=w70:path)
        n20 = Build Path(base path=w35, name or relative path="IconFolder.txt") -> (appended path=w43:path)
        n21 = Path To String(path=w53) -> (string=w72:string)
        n22 = Read from Text File(file (use dialog)=w43) -> (text=w37:string)  [unwired: 3 in, 3 out]
        n23 = Path To String(path=w65) -> (string=w63:string)
        n24 = Path To String(path=w67) -> (string=w64:string)
        n25 = Path To String(path=w70) -> (string=w71:string)
        n26 = call <vilib>:"Trim Whitespace.vi"("string"=w37) -> ("trimmed string"=w47:string)  [unwired: 1 in]
        n27 = Build Array(w63, w64, w71, w72) -> (w29:string[])
        n28 = Spreadsheet String To Array(delimiter (Tab)="\n", format string="%s", spreadsheet string=w47, array type (2D Dbl)=string[] []) -> (array=w66:string[])
        n29 = Build Array (concatenate)(w29, w66) -> (w30:string[])
        n30 = String To Path(string=w30) -> (path=w31:path[])
        n31 = for {
          tunnel: w31 -> [w78] mode=indexing
          shift-right: [w83] -> w46
          shift-left: path[] [] -> [w79]
          shift-right: [w82] -> w49
          shift-left: string[] [] -> [w81]
          tunnel: w30 -> [w80] mode=indexing
          n32 = Empty String/Path?(string/path=w78) -> (empty?=w76:bool)
          n33 = Search 1D Array(1D array=w79, element=w78) -> (index of element=w77:i32)  [unwired: 1 in]
          n34 = Greater Or Equal To 0?(x=w77) -> (x >= 0?=w75:bool)
          n35 = Or(x=w76, y=w75) -> (x .or. y?=w74:bool)
          n36 = case shown="False" w74 {
            tunnel: w78 -> [w87 _]
            tunnel: w79 -> [w90 w100]
            tunnel: [w89 w100] -> w83
            tunnel: w81 -> [w85 w99]
            tunnel: [w86 w99] -> w82
            tunnel: w80 -> [w84 _]
            frame False {
              n37 = call <vilib>:"Check if File or Folder Exists.vi"("path"=w87) -> ("file or folder exists?"=w88:bool)  [unwired: 8 in, 2 out]
              n38 = case shown="True" w88 {
                tunnel: w90 -> [w92 w98]
                tunnel: [w92 w97] -> w89
                tunnel: w87 -> [_ w96]
                tunnel: w85 -> [w91 w94]
                tunnel: [w91 w95] -> w86
                tunnel: w84 -> [_ w93]
                frame False {
                }
                frame True {
                  n39 = Build Array (concatenate)(w98, w96) -> (w97:path[])
                  n40 = Build Array (concatenate)(w94, w93) -> (w95:string[])
                }
              }
            }
            frame True {
            }
          }
        }
        n41 = Bundle By Name(cluster=w32, "Folders"=w46) -> (w33:T9)
        n42 = Build Array (concatenate)("<All icons>" ("y"), w49) -> (w42:string[])
        n43 = property on="_Folders" class="Ring (strict)"("Strings []"=w42, "Value"=0) -> ()  [unwired: 2 in, 2 out]
      }
      frame "ReadIcons" {
        n44 = local read "_Folders"() -> (w101:u16)
        n45 = Unbundle By Name(w102) -> ("Folders"=w105:path[])
        n46 = case shown="Default" w101 {
          selector: w101 -> [_ w113]
          tunnel: w105 -> [w112 w117]
          tunnel: [w112 w114] -> w106
          frame 0 {
            (unwired) 0 ("index")
          }
          frame Default {
            n47 = Decrement(x=w113) -> (x-1=w116:u16)
            n48 = Index Array(array=w117, index=w116) -> (element=w115:path)
            n49 = Build Array(w115) -> (w114:path[])
          }
        }
        n50 = call <vilib>:"Set Busy.vi"() -> ("error out"=w107:errorcluster)  [unwired: 10 in, 1 out]
        n51 = for {
          tunnel: w106 -> [w122] mode=indexing
          shift-right: [w118] -> w109
          shift-left: cluster{i32, "path out":path}[] [] -> [w119]
          shift-right: [w123] -> _
          shift-left: w107 -> [w120]
          n52 = call <vilib>:"Check if File or Folder Exists.vi"("path"=w122) -> ("file or folder exists?"=w121:bool)  [unwired: 8 in, 2 out]
          n53 = case shown="True" w121 {
            tunnel: [w125 w131] -> w123
            tunnel: w120 -> [w125 w130]
            tunnel: w122 -> [_ w129]
            tunnel: w119 -> [w124 w126]
            tunnel: [w124 w128] -> w118
            frame False {
            }
            frame True {
              n54 = call <vilib>:"Recursive File List.vi"("pattern"="*.png", "error in (no error)"=w130, "Folder Path"=w129) -> ("error out"=w133:errorcluster, "All Files in Dir"=w134:path[])  [unwired: 4 in, 3 out]
              n55 = for {
                tunnel: w134 -> [w142] mode=indexing
                tunnel: [w140] -> w127 mode=indexing
                shift-right: [w139] -> w131
                shift-left: w133 -> [w143]
                n56 = File/Directory Info(path=w142, error in=w143) -> (path out=w141:path, size=w138:i64, error out=w139:errorcluster)  [unwired: 4 out]
                n57 = Divide(x=w138, y=i64 100) -> (x/y=w136:dbl)
                n58 = To Long Integer(number=w136) -> (32bit integer=w135:i32)
                n59 = Bundle(w135, "path out"=w141) -> (w140:cluster{i32, "path out":path})  [unwired: 1 in]
              }
              n60 = Build Array (concatenate)(w126, w127) -> (w128:cluster{i32, "path out":path}[])
            }
          }
        }
        n61 = Sort 1D Array(array=w109) -> (sorted array=w104:cluster{i32, "path out":path}[])
        n62 = Bundle By Name(cluster=w102, "IconPaths"=w104) -> (w103:T9)
      }
      frame "DrawIcons" {
        w154 = 0  # IconsPerRow
        w150 = 10  # Border
        w152 = 15  # Gap
        # "Y"
        # "X"
        n63 = Unbundle By Name(w147) -> ("IconPaths"=w164:cluster{i32, "path out":path}[])
        n64 = local read "_IconSearchText"() -> (w165:string)
        n65 = property on="Icons" class="Pict"() -> ("Draw Area Size"=w157:T12)  [unwired: 2 in, 2 out]
        n66 = Unbundle By Name(w157) -> ("Width"=w151:u32)
        n67 = property on="Icons" class="Pict"("Origin"=T10 {"Horizontal"=0, "Vertical"=0}) -> ()  [unwired: 2 in, 2 out]
        n68 = call <vilib>:"Trim Whitespace.vi"("string"=w165) -> ("trimmed string"=w166:string)  [unwired: 1 in]
        n69 = for {
          shift-right: [w196] -> w145
          shift-left: w144 -> [w179]
          shift-right: [w183] -> _
          shift-left: w150 -> [w191]
          shift-right: [w194] -> w146
          shift-left: picture data[5B] ("new picture") -> [w195]
          shift-right: [w192] -> w158
          shift-left: T7[] [] -> [w193]
          shift-right: [w184] -> _
          shift-left: w154 -> [w185]
          shift-right: [w182] -> _
          shift-left: w150 -> [w186]
          shift-right: [w187] -> _
          shift-left: TRUE -> [w190]
          tunnel: w152 -> [w189]
          tunnel: w151 -> [w188]
          tunnel: w150 -> [w181]
          tunnel: w164 -> [w180] mode=indexing
          shift-right: [w178] -> w160
          shift-left: cluster{i32, i32, i32, i32}[] [] -> [w177]
          shift-right: [w175] -> w163
          shift-left: string[] [] -> [w176]
          tunnel: w166 -> [w174]
          n70 = Unbundle(w180) -> (w172:i32, "path out"=w173:path)
          n71 = case shown="Default" w174 {
            selector: w174 -> [w202 _]
            tunnel: w173 -> [w203 _]
            tunnel: [w197 TRUE] -> w169
            frame Default {
              n72 = To Lower Case(string=w202) -> (all lower case string=w199:string)
              n73 = call <vilib>:"Get File Extension.vi"("file"=w203) -> ("filename without extension"=w201:string)  [unwired: 6 in, 4 out]
              n74 = To Lower Case(string=w201) -> (all lower case string=w200:string)
              n75 = Match Pattern(string=w200, regular expression=w199) -> (offset past match=w198:i32)  [unwired: 1 in, 3 out]
              n76 = Greater Or Equal To 0?(x=w198) -> (x >= 0?=w197:bool)
            }
            frame "" {
            }
          }
          n77 = Less Or Equal?(x=w172, y=50) -> (x <= y?=w170:bool)
          n78 = And(x=w169, y=w170) -> (x .and. y?=w168:bool)
          n79 = case shown="True" w168 {
            tunnel: w173 -> [_ w217]
            tunnel: w179 -> [w213 w246]
            tunnel: [w213 w245] -> w196
            tunnel: w195 -> [w212 w244]
            tunnel: [w212 w223] -> w194
            tunnel: w193 -> [w211 w229]
            tunnel: [w211 w243] -> w192
            tunnel: w191 -> [w209 w226]
            tunnel: w190 -> [w207 w242]
            tunnel: w189 -> [_ w228]
            tunnel: w188 -> [_ w239]
            tunnel: [w207 w238] -> w187
            tunnel: w186 -> [w208 w233]
            tunnel: w185 -> [w210 w232]
            tunnel: [w210 w231] -> w184
            tunnel: [w209 w221] -> w183
            tunnel: [w208 w225] -> w182
            tunnel: w181 -> [_ w227]
            tunnel: w177 -> [w206 w220]
            tunnel: [w206 w219] -> w178
            tunnel: w176 -> [w205 w215]
            tunnel: [w205 w216] -> w175
            frame False {
            }
            frame True {
              # "Place This Icon on a new row"
              n80 = call <vilib>:"Read PNG File.vi"("error in (no error)"=w246, "path to PNG file"=w217) -> ("error out"=w245:errorcluster, "image data"=w237:T7)  [unwired: 7 in, 1 out]
              n81 = Unbundle By Name(w237) -> ("Rectangle"=w236:T13)
              n82 = Unbundle By Name(w237) -> ("Rectangle.right"=w224:i16)
              n83 = Select(t=0, s=w242, f=w228) -> (s? t:f=w241:i32)
              n84 = Add(x=w241, y=w226) -> (x+y=w234:i32)
              n85 = Strip Path(path=w217) -> (name=w214:string)  [unwired: 1 out]
              n86 = Add(x=w234, y=w224) -> (x+y=w230:i32)
              n87 = Greater?(x=w230, y=w239) -> (0:w238:bool)
              n88 = Build Array (concatenate)(w229, w237) -> (w243:T7[])
              n89 = case shown="True" w238 {
                tunnel: [w251 w257] -> w235
                tunnel: w234 -> [w248 _]
                tunnel: w233 -> [w247 w252]
                tunnel: w232 -> [w250 w260]
                tunnel: [w249 1] -> w231
                tunnel: w229 -> [_ w261]
                tunnel: w228 -> [_ w255]
                tunnel: w227 -> [_ w254]
                tunnel: w226 -> [_ _]
                tunnel: [w247 w253] -> w225
                tunnel: w224 -> [_ _]
                frame False {
                  n90 = Bundle(w248, "Border"=w247, w248, "Border"=w247) -> (w251:cluster{i32, "Border":i32, i32, "Border":i32})  [unwired: 1 in]
                  n91 = Increment(x=w250) -> (x+1=w249:i32)
                }
                frame True {
                  n92 = Delete From Array(array=w261, length=w260) -> (deleted portion=w259:T7[])  [unwired: 1 in, 1 out]
                  n93 = for {
                    tunnel: w259 -> [w264] mode=indexing
                    tunnel: [w263] -> w258 mode=indexing
                    n94 = Unbundle By Name(w264) -> ("Rectangle.bottom"=w263:i16)
                  }
                  n95 = Array Max & Min(array=w258) -> (max value=w256:i16)  [unwired: 3 out]
                  n96 = Compound Arithmetic op=ADD(w252, w255, w256) -> (w253:i32)
                  n97 = Bundle("Border"=w254, w253, "Border"=w254, w253) -> (w257:cluster{"Border":i32, i32, "Border":i32, i32})  [unwired: 1 in]
                }
              }
              n98 = Add(x=w235, y=w236) -> (x+y=w218:cluster{i32, i32, i32, i32})
              n99 = Bundle By Name(cluster=w237, "Rectangle"=w218) -> (w222:T7)
              n100 = Build Array (concatenate)(w220, w218) -> (w219:cluster{i32, i32, i32, i32}[])
              n101 = Build Array (concatenate)(w215, w214) -> (w216:string[])
              n102 = Unbundle By Name(w222) -> ("Rectangle.right"=w221:i16)
              n103 = call <vilib>:"Draw Flattened Pixmap.vi"("image data"=w222, "picture"=w244) -> ("new picture"=w223:picture)  [unwired: 7 in]
            }
          }
        }
        "Icons" <- w146
        n104 = property on="DragIcon" class="Pict"("Visible"=FALSE) -> ()  [unwired: 2 in, 2 out]
        n105 = Bundle By Name(cluster=w147, "Icons"=w158, "IconPos"=w160, "IconNames"=w163) -> (w148:T9)
      }
      frame "SetBusy", "UnsetBusy" {
        n106 = case shown="\"UnsetBusy\", Default" w265 {
          frame "UnsetBusy", Default {
            n107 = call <vilib>:"Unset Busy.vi"() -> ()  [unwired: 11 in, 1 out]
          }
          frame "SetBusy" {
            n108 = call <vilib>:"Set Busy.vi"() -> ()  [unwired: 10 in, 2 out]
          }
        }
      }
      frame "", "Idle" {
        n109 = event shown="[4] \"Icons\", \"DragIcon\": Mouse Move" {
          selector: _ -> [_ _ _ _ _ _ _ _ _ _ _ _ _ _ _ _ _]
          dyn-events: _ -> [_ _ _ _ _ _ _ _ _ _ _ _ _ _ _ _ _]
          timeout: _ -> [_ _ _ _ _ _ _ _ _ _ _ _ _ _ _ _ _]
          tunnel: w273 -> [w275 w278 w281 w285 w288 w325 w380 w389 w398 w403 w404 w447 w453 w507 w522 w526 w531]
          tunnel: [w275 w278 w281 w285 w289 w326 w381 w390 w396 w401 w405 w448 w454 w508 w522 w527 w532] -> w272
          tunnel: w271 -> [w274 w277 w280 w284 w292 w343 w384 w393 w397 w402 w411 w450 w464 w521 w524 w529 w536]
          tunnel: [w274 w277 w280 w284 w292 w343 w384 w393 w397 w402 w411 w450 w464 w521 w524 w529 w536] -> w270
          tunnel: [_ "DrawIcons" "SetBusy\nReadIcons\nDrawIcons\nUnsetBusy" w282 w287 w324 _ _ "Exit" ("t") "Exit" ("t") w406 _ w452 "GetImageData\nUpdateIcon" ("y") _ _ "UpdateIcon" ("y")] -> w269
          event Timeout {
            n110 = event-data() -> ()  [unwired: 1 in, 1 out]
          }
          event "_IconSearchText": Value Change {
            n111 = event-data() -> ()  [unwired: 1 in, 6 out]
          }
          event "_Folders": Value Change {
            n112 = event-data() -> ()  [unwired: 1 in, 6 out]
          }
          event "_Manage": Value Change {
            n113 = event-data() -> ()  [unwired: 1 in, 6 out]
            n114 = call <resource>:"GDSLvIcon_ManageIconFolderDialog.vi"() -> ("Cancelled"=w283:bool)  [unwired: 10 in, 1 out]
            n115 = case shown="False" w283 {
              tunnel: ["SetBusy\nUpdateIconFolderList\nReadIcons\nDrawIcons\nUnsetBusy" _] -> w282
              frame False {
              }
              frame True {
              }
            }
          }
          event "Icons", "DragIcon": Mouse Move {
            n116 = event-data() -> ("Coords"=w290:T8)  [unwired: 1 in]
            n117 = Unbundle By Name(w288) -> ("DraggingIcon"=w291:bool)
            n118 = case shown="False" w291 {
              tunnel: w288 -> [w305 w323]
              tunnel: [w304 w323] -> w289
              tunnel: [w302 "Idle" ("t")] -> w287
              tunnel: w290 -> [w301 _]
              tunnel: w288 -> [w298 _]
              frame False {
                n119 = property on="Icons" class="Pict"() -> ("Origin"=w297:T10, "Position"=w293:T11)  [unwired: 2 in, 2 out]
                n120 = Unbundle By Name(w298) -> ("IconPos"=w306:T14)
                n121 = Subtract(x=w301, y=w293) -> (x-y=w296:T8)
                n122 = Add(x=w297, y=w296) -> (x+y=w295:T8)
                n123 = for {
                  tunnel: w306 -> [w316] mode=indexing
                  tunnel: w295 -> [w318]
                  tunnel: [w308] -> w303
                  tunnel: [w307] -> w300
                  i -> [w307]
                  stop <- w308 stop-if-true
                  n124 = Unbundle(w316) -> ("left"=w315:i16, "top"=w311:i16, "right"=w314:i16, "bottom"=w313:i16)
                  n125 = Unbundle(w318) -> ("Horizontal"=w317:i32, "Vertical"=w312:i32)
                  n126 = In Range and Coerce(upper limit=w314, x=w317, lower limit=w315) -> (In Range?=w309:bool)  [unwired: 1 out]
                  n127 = In Range and Coerce(upper limit=w313, x=w312, lower limit=w311) -> (In Range?=w310:bool)  [unwired: 1 out]
                  n128 = And(x=w309, y=w310) -> (x .and. y?=w308:bool)
                }
                n129 = Select(t=w300, s=w303, f=-1) -> (s? t:f=w294:i32)
                n130 = case shown="True" w303 {
                  tunnel: ["Idle" ("t") "ShowDragIcon" ("t")] -> w302
                  frame False {
                    n131 = property on="DragIcon" class="Pict"("Visible"=FALSE) -> ()  [unwired: 2 in, 2 out]
                  }
                  frame True {
                  }
                }
                n132 = Bundle By Name(cluster=w305, "IconSelected"=w294) -> (w304:T9)
              }
              frame True {
              }
            }
          }
          event "_IconPreview": Mouse Down {
            w340 = 4 ("y")
            n133 = event-data() -> ("Coords"=w327:T8)  [unwired: 1 in]
            n134 = property on="_IconPreview" class="Pict"() -> ("Mouse"=w336:T15)  [unwired: 2 in, 2 out]
            n135 = Unbundle By Name(w336) -> ("Mouse Position.X"=w339:i32, "Mouse Position.Y"=w337:i32)
            n136 = Unbundle By Name(w325) -> ("IconDropped"=w328:i32, "TextBounds"=w329:T16)
            n137 = Unbundle(w329) -> ("FirstRow"=w331:i32, "FirstColumn"=w332:i32, "LastRow"=w330:i32, "LastColumn"=w335:i32)
            n138 = Divide(x=w339, y=w340) -> (x/y=w341:dbl)
            n139 = Divide(x=w337, y=w340) -> (x/y=w338:dbl)
            n140 = In Range and Coerce(upper limit=w330, x=w338, lower limit=w331) -> (In Range?=w333:bool)  [unwired: 1 out]
            n141 = In Range and Coerce(upper limit=w335, x=w341, lower limit=w332) -> (In Range?=w334:bool)  [unwired: 1 out]
            n142 = And(x=w333, y=w334) -> (x .and. y?=w342:bool)
            n143 = case shown="False" w342 {
              tunnel: w325 -> [w348 w379]
              tunnel: [w347 w376] -> w326
              tunnel: [w346 "Idle" ("y")] -> w324
              tunnel: w327 -> [w345 w370]
              tunnel: w328 -> [w344 _]
              tunnel: w325 -> [_ w374]
              frame False {
                n144 = case shown="0.." w344 {
                  selector: w344 -> [_ w351]
                  tunnel: w348 -> [w350 w366]
                  tunnel: [w350 w365] -> w347
                  tunnel: ["Idle" ("y") "ShowDragIcon\nUpdateIcon" ("y")] -> w346
                  tunnel: w345 -> [_ w352]
                  frame Default {
                  }
                  frame 0.. {
                    n145 = property on="DragIcon" class="Pict"() -> ("Draw Area Size"=w363:T12)  [unwired: 2 in, 2 out]
                    n146 = Divide(x=w363, y=2) -> (x/y=w361:cluster{"Width":dbl, "Height":dbl})
                    n147 = property on="_IconPreview" class="Pict"() -> ("Position"=w359:T11)  [unwired: 2 in, 2 out]
                    n148 = Subtract(x=w352, y=w361) -> (x-y=w355:cluster{dbl, dbl})
                    n149 = property on="DragIcon" class="Pict"("Position"=w355) -> ()  [unwired: 2 in, 2 out]
                    n150 = Add(x=w359, y=T11 {"Left"=0, "Top"=16}) -> (x+y=w358:T11)
                    n151 = Subtract(x=w355, y=w358) -> (x-y=w356:cluster{dbl, dbl})
                    n152 = Divide(x=w356, y=u8 4 ("Disabled")) -> (x/y=w354:cluster{dbl, dbl})
                    n153 = Bundle By Name(cluster=w366, "IconSelected"=w351, "DraggingIcon"=TRUE ("Draging"), "BgIconOffset"=w354) -> (w365:T9)
                  }
                }
              }
              frame True {
                n154 = Unbundle By Name(w374) -> ("IconInfo.Offset.X"=w373:i32, "IconInfo.Offset.Y"=w372:i32)
                n155 = Bundle("X"=w373, "Y"=w372) -> (w368:cluster{"X":i32, "Y":i32})  [unwired: 1 in]
                n156 = Multiply(x=w368, y=4) -> (x*y=w367:cluster{"X":i32, "Y":i32})
                n157 = Subtract(x=w370, y=w367) -> (x-y=w369:T8)
                n158 = Bundle By Name(cluster=w379, "DraggingIcon"=FALSE, "DraggingText"=TRUE, "StartTextDraggingPos"=w369) -> (w376:T9)
              }
            }
          }
          event "_IconPreview": Mouse Enter {
            n159 = event-data() -> ()  [unwired: 1 in, 4 out]
            n160 = Unbundle By Name(w380) -> ("DraggingIcon"=w383:bool, "IconDropped"=w382:i32)
            n161 = case shown="False" w383 {
              tunnel: w380 -> [w387 w388]
              tunnel: [w386 w388] -> w381
              tunnel: w382 -> [w385 _]
              frame False {
                n162 = Bundle By Name(cluster=w387, "IconSelected"=w385) -> (w386:T9)
              }
              frame True {
              }
            }
          }
          event "_IconPreview": Mouse Up {
            w391 = FALSE ("Draging")
            n163 = event-data() -> ()  [unwired: 1 in, 8 out]
            n164 = Unbundle By Name(w389) -> ("IconSelected"=w392:i32)
            n165 = Bundle By Name(cluster=w389, "IconDropped"=w392, "Moving"=w391, "DraggingIcon"=w391) -> (w390:T9)
            n166 = property on="DragIcon" class="Pict"("Visible"=w391) -> ()  [unwired: 2 in, 2 out]
          }
          event "Accept", "_Cancel": Value Change {
            n167 = event-data() -> ()  [unwired: 1 in, 6 out]
            n168 = Bundle By Name(cluster=w398, "Cancelled"="_Cancel") -> (w396:T9)
          }
          event Panel Close? {
            w399 = TRUE ("Cancelled")
            n169 = event-data() -> ()  [unwired: 1 in, 4 out]
            n170 = Bundle By Name(cluster=w403, "Cancelled"=w399) -> (w401:T9)
            n171 = event-data("Discard?"=w399) -> ()  [unwired: 1 in, 1 out]
          }
          event Mouse Move {
            n172 = event-data() -> ("Coords"=w407:T8)  [unwired: 1 in]
            n173 = Unbundle By Name(w404) -> ("StartTextDraggingPos"=w410:T8)
            n174 = Unbundle By Name(w404) -> ("DraggingText"=w409:bool, "DraggingIcon"=w408:bool)
            n175 = case shown="False" w408 {
              tunnel: w404 -> [w417 w439]
              tunnel: [w416 w438] -> w405
              tunnel: w407 -> [w413 w434]
              tunnel: w404 -> [w412 _]
              tunnel: [w415 "UpdateIcon" ("y")] -> w406
              tunnel: w409 -> [w418 _]
              tunnel: w410 -> [w414 _]
              frame False {
                n176 = case shown="True" w418 {
                  tunnel: w417 -> [w419 w432]
                  tunnel: [w419 w431] -> w416
                  tunnel: [_ "Generate icon"] -> w415
                  tunnel: w414 -> [_ w428]
                  tunnel: w413 -> [_ w429]
                  tunnel: w412 -> [_ w427]
                  frame False {
                  }
                  frame True {
                    n177 = Subtract(x=w429, y=w428) -> (x-y=w424:T8)
                    n178 = Unbundle By Name(w427) -> ("IconInfo.Offset"=w422:cluster{"X":i32, "Y":i32})
                    n179 = Divide(x=w424, y=u8 4 ("f")) -> (x/y=w423:cluster{"Horizontal":dbl, "Vertical":dbl})
                    n180 = Unbundle By Name(w423) -> ("Horizontal"=w421:dbl, "Vertical"=w420:dbl)
                    n181 = Bundle By Name(cluster=w432, "OldOffset"=w422) -> (w426:T9)
                    n182 = Bundle By Name(cluster=w426, "IconInfo.Offset.X"=w421, "IconInfo.Offset.Y"=w420) -> (w431:T9)
                  }
                }
              }
              frame True {
                n183 = property on="DragIcon" class="Pict"() -> ("Draw Area Size"=w444:T12)  [unwired: 2 in, 2 out]
                n184 = property on="_IconPreview" class="Pict"() -> ("Position"=w442:T11)  [unwired: 2 in, 2 out]
                n185 = Divide(x=w444, y=2.0 ("Waveform Chart")) -> (x/y=w445:cluster{"Width":dbl, "Height":dbl})
                n186 = Add(x=w442, y=T11 {"Left"=0, "Top"=16}) -> (x+y=w441:T11)
                n187 = Subtract(x=w434, y=w445) -> (x-y=w433:cluster{dbl, dbl})
                n188 = Subtract(x=w433, y=w441) -> (x-y=w436:cluster{dbl, dbl})
                n189 = property on="DragIcon" class="Pict"("Position"=w433) -> ()  [unwired: 2 in, 2 out]
                n190 = Divide(x=w436, y=u8 4 ("Disabled")) -> (x/y=w435:cluster{dbl, dbl})
                n191 = Bundle By Name(cluster=w439, "BgIconOffset"=w435) -> (w438:T9)
              }
            }
          }
          event Mouse Up; Mouse Leave {
            w449 = FALSE ("DraggingText")
            n192 = event-data() -> ()  [unwired: 1 in, 4 out]
            n193 = Bundle By Name(cluster=w447, "DraggingText"=w449) -> (w448:T9)
            n194 = property on="DragIcon" class="Pict"("Visible"=w449) -> ()  [unwired: 2 in, 2 out]
          }
          event Key Down? {
            n195 = event-data() -> ("VKey"=w451:T17, "PlatMods"=w458:T18)  [unwired: 1 in]
            n196 = property on="_Folders" class="Ring (strict)"() -> ("Key Focus"=w455:bool)  [unwired: 2 in, 2 out]
            n197 = property on="_IconSearchText" class="Str"() -> ("Key Focus"=w456:bool)  [unwired: 2 in, 2 out]
            n198 = Unbundle By Name(w453) -> ("IconInfo.Offset.X"=w461:i32, "IconInfo.Offset.Y"=w460:i32)
            n199 = Compound Arithmetic op=AND(invert w456, invert w455) -> (w457:bool)
            n200 = Unbundle By Name(w458) -> ("Ctrl"=w462:bool)
            n201 = Or(x=w462, y=w457) -> (x .or. y?=w463:bool)
            n202 = case shown="False" w463 {
              tunnel: w453 -> [w466 w470]
              tunnel: [w466 w474] -> w454
              tunnel: w451 -> [_ w473]
              tunnel: w460 -> [_ w467]
              tunnel: w461 -> [_ w468]
              tunnel: ["Idle" w472] -> w452
              tunnel: [_ w471] -> w459
              frame False {
              }
              frame True {
                n203 = Bundle By Name(cluster=w470, "OldOffset.X"=w468, "OldOffset.Y"=w467) -> (w469:T9)
                n204 = case shown="Default" w473 {
                  tunnel: w469 -> [w481 w483 w490 w497 w504]
                  tunnel: [w480 w483 w489 w496 w503] -> w474
                  tunnel: w467 -> [w479 _ w488 w494 w501]
                  tunnel: w468 -> [w477 _ w486 w495 w502]
                  tunnel: ["Generate icon" "Idle" "Generate icon" "Generate icon" "Generate icon"] -> w472
                  tunnel: [TRUE _ TRUE TRUE TRUE] -> w471
                  frame "Up" {
                    n205 = Decrement(x=w479) -> (x-1=w478:i32)
                    n206 = Bundle By Name(cluster=w481, "IconInfo.Offset.X"=w477, "IconInfo.Offset.Y"=w478) -> (w480:T9)
                  }
                  frame Default {
                  }
                  frame "Down" {
                    n207 = Increment(x=w488) -> (x+1=w487:i32)
                    n208 = Bundle By Name(cluster=w490, "IconInfo.Offset.X"=w486, "IconInfo.Offset.Y"=w487) -> (w489:T9)
                  }
                  frame "Left" {
                    n209 = Decrement(x=w495) -> (x-1=w493:i32)
                    n210 = Bundle By Name(cluster=w497, "IconInfo.Offset.X"=w493, "IconInfo.Offset.Y"=w494) -> (w496:T9)
                  }
                  frame "Right" {
                    n211 = Increment(x=w502) -> (x+1=w500:i32)
                    n212 = Bundle By Name(cluster=w504, "IconInfo.Offset.X"=w500, "IconInfo.Offset.Y"=w501) -> (w503:T9)
                  }
                }
              }
            }
            n213 = event-data("Discard?"=w459) -> ()  [unwired: 1 in, 1 out]
          }
          event "DragIcon": Mouse Down {
            n214 = event-data() -> ("Coords"=w506:T8)  [unwired: 1 in]
            n215 = property on="DragIcon" class="Pict"() -> ("Draw Area Size"=w510:T12)  [unwired: 2 in, 2 out]
            n216 = Divide(x=w510, y=2) -> (x/y=w512:cluster{"Width":dbl, "Height":dbl})
            n217 = property on="_IconPreview" class="Pict"() -> ("Position"=w514:T11)  [unwired: 2 in, 2 out]
            n218 = Subtract(x=w506, y=w512) -> (x-y=w518:cluster{dbl, dbl})
            n219 = Add(x=w514, y=T11 {"Left"=0, "Top"=16}) -> (x+y=w515:T11)
            n220 = Subtract(x=w518, y=w515) -> (x-y=w517:cluster{dbl, dbl})
            n221 = Divide(x=w517, y=u8 4 ("Disabled")) -> (x/y=w519:cluster{dbl, dbl})
            n222 = property on="DragIcon" class="Pict"("Position"=w518, "Visible"=TRUE) -> ()  [unwired: 2 in, 2 out]
            n223 = Bundle By Name(cluster=w507, "DraggingIcon"=TRUE ("Draging"), "BgIconOffset"=w519) -> (w508:T9)
          }
          event "DragIcon": Mouse Leave {
            n224 = event-data() -> ()  [unwired: 1 in, 4 out]
            n225 = Unbundle By Name(w522) -> ("DraggingIcon"=w523:bool)
            n226 = case shown="True" w523 {
              selector: w523 -> [w525 _]
              frame False {
                n227 = property on="DragIcon" class="Pict"("Visible"=w525) -> ()  [unwired: 2 in, 2 out]
              }
              frame True {
              }
            }
          }
          event "DragIcon": Mouse Up {
            w528 = FALSE ("Draging")
            n228 = event-data() -> ()  [unwired: 1 in, 8 out]
            n229 = Bundle By Name(cluster=w526, "DraggingIcon"=w528) -> (w527:T9)
            n230 = property on="DragIcon" class="Pict"("Visible"=w528) -> ()  [unwired: 2 in, 2 out]
          }
          event "FloodFillMask": Value Change {
            n231 = event-data() -> ()  [unwired: 1 in, 6 out]
            n232 = Unbundle By Name(w531) -> ("BgIcon"=w534:u8[][])
            n233 = call <resource>:"GDSIconEditor_CreateImageMask.vi"("Flood Fill"="FloodFillMask", "8-bit pixmap"=w534) -> ("Array"=w535:u8[])
            n234 = Bundle By Name(cluster=w531, "BgIconMask"=w535) -> (w532:T9)
          }
        }
      }
      frame "GetImageData" {
        # "Create White mask Color, When Mouse Down"
        n235 = Unbundle By Name(w538) -> ("Icons"=w540:T7[], "IconSelected"=w541:i32)
        n236 = Index Array(array=w540, index=w541) -> (element=w547:T7)
        n237 = call <resource>:"GDSIconEditor_ShrinkImage.vi"("image data"=w547) -> ("image subset"=w546:T7)  [unwired: 9 in]
        n238 = call <resource>:"GDSIconEditor_ImageDataTo8Bit.vi"("image data"=w546) -> ("NoMaskFound"=w545:bool, "8-bit pixmap"=w544:u8[][], "mask"=w542:u8[])  [unwired: 7 in, 1 out]
        n239 = call <vilib>:"Draw Flattened Pixmap.vi"("image data"=w546) -> ("new picture"=→"DragIcon":picture)  [unwired: 8 in]
        n240 = property on="FloodFillMask" class="Bool (strict)"("Visible"=w545) -> ()  [unwired: 2 in, 2 out]
        n241 = case shown="True" w545 {
          tunnel: w544 -> [_ w553]
          tunnel: w542 -> [w550 _]
          tunnel: [w550 w552] -> w543
          frame False {
          }
          frame True {
            n242 = local read "FloodFillMask"() -> (w551:bool)
            n243 = call <resource>:"GDSIconEditor_CreateImageMask.vi"("Flood Fill"=w551, "8-bit pixmap"=w553) -> ("Array"=w552:u8[])
          }
        }
        n244 = Bundle By Name(cluster=w538, "BgIcon"=w544, "BgIconMask"=w543) -> (w539:T9)
      }
      frame "ShowDragIcon" {
        w572 = 2.0 ("Waveform Chart")
        w583 = 4 ("x")
        n245 = Unbundle By Name(w560) -> ("IconNames"=w591:string[], "Icons"=w561:T7[], "IconSelected"=w592:i32, "IconPos"=w564:T14)
        n246 = property on="Icons" class="Pict"() -> ("Origin"=w559:T10, "Position"=w558:T11)  [unwired: 2 in, 2 out]
        n247 = Index Array(array=w591, index=w592) -> (element=→"_IconName":string)
        n248 = Index Array(array=w561, index=w592) -> (element=w594:T7)
        n249 = Index Array(array=w564, index=w592) -> (element=w565:T13)
        n250 = Unbundle By Name(w565) -> ("left"=w566:i16, "top"=w570:i16, "right"=w567:i16, "bottom"=w569:i16)
        n251 = call <resource>:"GDSIconEditor_ShrinkImage.vi"("image data"=w594) -> ("image subset"=w595:T7)  [unwired: 9 in]
        n252 = Unbundle By Name(w595) -> ("Rectangle.right"=w587:i16, "Rectangle.bottom"=w586:i16)
        n253 = call <vilib>:"Draw Flattened Pixmap.vi"("image data"=w595) -> ("new picture"=w581:picture)  [unwired: 8 in]
        n254 = Add(x=w570, y=w569) -> (x+y=w571:i16)
        n255 = Add(x=w566, y=w567) -> (x+y=w568:i16)
        n256 = Divide(x=w571, y=w572) -> (x/y=w574:dbl)
        n257 = Divide(x=w568, y=w572) -> (x/y=w573:dbl)
        n258 = Subtract(x=w558, y=w559) -> (x-y=w590:T11)
        n259 = Bundle("right"=w587, "bottom"=w586) -> (w582:cluster{"right":i16, "bottom":i16})  [unwired: 1 in]
        n260 = Bundle(w573, w574) -> (w575:cluster{dbl, dbl})  [unwired: 1 in]
        n261 = Increment(x=w582) -> (x+1=w563:cluster{"right":i16, "bottom":i16})
        n262 = Add(x=w575, y=w590) -> (x+y=w576:cluster{dbl, dbl})
        n263 = Divide(x=w563, y=2.0 ("Waveform Chart")) -> (x/y=w584:cluster{"right":dbl, "bottom":dbl})
        n264 = Multiply(x=w583, y=w584) -> (x*y=w585:cluster{"right":dbl, "bottom":dbl})
        n265 = Subtract(x=w576, y=w585) -> (x-y=w589:cluster{dbl, dbl})
        n266 = Multiply(x=w583, y=w587) -> (x*y=w579:i32)
        n267 = Multiply(x=w583, y=w586) -> (x*y=w580:i32)
        n268 = Bundle(w579, w580) -> (w578:cluster{i32, i32})  [unwired: 1 in]
        n269 = Match Pattern(string=w557, regular expression="UpdateIcon" ("t")) -> (offset past match=w555:i32)  [unwired: 1 in, 3 out]
        n270 = Greater Or Equal To 0?(x=w555) -> (x >= 0?=w554:bool)
        n271 = property on="DragIcon" class="Pict"("Draw Area Size"=w578, "Value"=w581, "Visible"=TRUE) -> (error out=w588:errorcluster)  [unwired: 2 in, 1 out]
        n272 = case shown="False" w554 {
          tunnel: w588 -> [w598 _]
          tunnel: w589 -> [w597 _]
          frame False {
            n273 = property on="DragIcon" class="Pict"(error in=w598, "Position"=w597) -> ()  [unwired: 1 in, 2 out]
          }
          frame True {
          }
        }
      }
      frame "UpdateIcon" {
        w613 = T2 {"BgIcon"=[], "BgIconOffset"={"X"=0, "Y"=0}, "BgIconMask"=[], "ColorsOkayforiconToBeOnTopOf"=[]}  # BgIcon
        n274 = Unbundle By Name(w599) -> ("IconInfo.BodyBackgroundColor"=w601:u32, "IconInfo.RowStart(0)"=w602:i32, "IconInfo.ImageRows(32)"=w603:i32, "IconInfo.FrameColor"=w609:u32, "IconInfo.FrameThickness(1)"=w608:u32, "IconInfo.HeaderIcon"=w604:u8[][])
        n275 = Unbundle By Name(w599) -> ("BodyIcon"=w612:u8[][])
        n276 = Unbundle By Name(w599) -> ("BgIcon"=w614:u8[][], "BgIconOffset"=w615:cluster{"X":i32, "Y":i32}, "BgIconMask"=w617:u8[], "IconInfo.HeaderBackgroundColor"=w618:u32)
        n277 = call <resource>:"GDSLvIcon_Convert24bitTo8bitColor.vi"("Color 24bit In"=w618) -> ("Color out(256)"=w619:u8)  [unwired: 15 in, 3 out]
        n278 = call <resource>:"GDSLvIcon_Convert24bitTo8bitColor.vi"("Color 24bit In"=w601) -> ("Color out(256)"=w620:u8)  [unwired: 15 in, 3 out]
        n279 = Build Array(w619, w620) -> (w616:u8[])
        n280 = Bundle By Name(cluster=w613, "BgIcon"=w614, "BgIconOffset"=w615, "BgIconMask"=w617, "ColorsOkayforiconToBeOnTopOf"=w616) -> (w621:T2)
        n281 = call <resource>:"GDSLvIcon_CreateIconPicture.vi"("FrameColor"=w609, "FrameThickness(1)"=w608, "HeaderIconIn"=w604, "BodyIconIn"=w612, "error in (no error)"=w605, "ImageRows(32)"=w603, "BigSizeIcon(x6)"=4, "RowStart(0)"=w602, "BgIcon"=w621) -> ("WholeIconOut"=w622:u8[][], "IconPictureOut"=w610:picture, "LargeIconPictureOut(x6)"=w611:picture, "error out"=w606:errorcluster)  [unwired: 5 in, 2 out]
        n282 = Bundle By Name(cluster=w599, "IconInfo.CurrentIcon"=w621, "IconOut"=w622) -> (w600:T9)
        n283 = local write "_IconPreview"(w611) -> ()
        n284 = local write "_After"(w610) -> ()
      }
      frame "Generate icon" {
        n285 = Unbundle By Name(w635) -> ("IconInfo.RowStart(0)"=w640:i32, "IconInfo.ImageRows(32)"=w630:i32)
        n286 = Unbundle By Name(w635) -> ("IconInfo.FrameColor"=w634:u32, "IconInfo.FrameThickness(1)"=w633:u32, "IconInfo.BodyIconHeight"=w632:i32, "IconInfo.BodyIconWidth"=w631:i32)
        n287 = Unbundle By Name(w635) -> ("OldOffset.X"=w625:i32, "OldOffset.Y"=w653:i32, "IconInfo.CurrentIcon"=w629:T2)
        n288 = Unbundle By Name(w635) -> ("IconInfo.Offset"=w649:cluster{"X":i32, "Y":i32}, "IconInfo.HeaderIcon"=w641:u8[][], "IconInfo.IconTextDataType"=w628:T4, "IconInfo.BodyTextColor"=w627:u32, "IconInfo.BodyBackgroundColor"=w626:u32)
        n289 = Unbundle By Name(w649) -> ("X"=w650:i32, "Y"=w654:i32)
        n290 = call <resource>:"GDSLvIcon_GenerateIconText.vi"("Text"=w628, "TextPixelHeight(5-30)"=w632, "Foreground color"=w627, "Background color"=w626, "error in (no error)"=w636, "Offset"=w649, "Text Pixel width(32-FrameThicknes*2))"=w631) -> ("X-Limited"=w647:bool, "Y-Limited"=w651:bool, "TextOut"=w655:u8[][], "TextBounds"=w656:T16, "error out"=w644:errorcluster)  [unwired: 8 in]
        n291 = Select(t=w625, s=w647, f=w650) -> (s? t:f=w648:i32)
        n292 = Select(t=w653, s=w651, f=w654) -> (s? t:f=w652:i32)
        n293 = call <resource>:"GDSLvIcon_CreateIconPicture.vi"("FrameColor"=w634, "FrameThickness(1)"=w633, "HeaderIconIn"=w641, "BodyIconIn"=w655, "error in (no error)"=w644, "ImageRows(32)"=w630, "BigSizeIcon(x6)"=4, "RowStart(0)"=w640, "BgIcon"=w629) -> ("WholeIconOut"=w646:u8[][], "IconPictureOut"=w639:picture, "LargeIconPictureOut(x6)"=w638:picture, "BodyOffset"=w658:cluster{"X":i32, "Y":i32}, "error out"=w637:errorcluster)  [unwired: 5 in, 1 out]
        n294 = Unbundle(w658) -> ("X"=w661:i32, "Y"=w660:i32)
        n295 = Bundle("Y"=w660, "X"=w661, "Y"=w660, "X"=w661) -> (w659:cluster{"Y":i32, "X":i32, "Y":i32, "X":i32})  [unwired: 1 in]
        n296 = Add(x=w659, y=w656) -> (x+y=w657:cluster{i32, i32, i32, i32})
        n297 = Bundle By Name(cluster=w635, "IconInfo.Offset.X"=w648, "IconInfo.Offset.Y"=w652, "Icon exist"=TRUE, "IconOut"=w646, "BodyIcon"=w655, "TextBounds"=w657) -> (w642:T9)
        n298 = local write "_After"(w639) -> ()
        n299 = local write "_IconPreview"(w638) -> ()
      }
      frame "Error", "Exit", Default {
      }
    }
  }
  "error out" <- w10
  n300 = Unbundle By Name(w8) -> ("Cancelled"=→"Cancelled":bool, "IconInfo.CurrentIcon"=→"CurrentIcon":T2, "BodyIcon"=→"BodyIcon":u8[][], "IconInfo.Offset"=→"Offset":cluster{"X":i32, "Y":i32}, "Icon exist"=→"Icon exist":bool)
